vi "steuerprogramm.vi"() -> ()   [LabVIEW 2010]
uses:
  <vilib>/userDefined/High Color/nirio_resource_hc.ctl
  <vilib>/rvi/interface/nirviOpenFPGA/nirviOpenFPGA.xnode
  C:/Users/HAGAR-IV/Desktop/Zeugs/markus/version feb 2012/test/Auslesenkopiekopie2.vi
  <vilib>/rvi/interface/nirviMethod/nirviMethod.xnode
  <vilib>/rvi/interface/nirviReadWriteControl/nirviReadWriteControl.xnode
  <vilib>/rvi/errors/niLvFpgaWhatHappensToTopLevelVI.ctl
  <vilib>/rvi/interface/common/niFpgaNodeNameForErrorReporting.ctl
  <vilib>/rvi/errors/niLvFpgaAdjustHostInterfaceError.vi
  gvbooleschRT.vi
  <vilib>/functionblocks/FB Core/FB Core.xnode
  <vilib>/functionblocks/Counter/Elapsed Timer/Elapsed Timer.vi
  <vilib>/functionblocks/NI_FunctionBlock Libraries.lvlib
  <vilib>/rvi/interface/nirviCloseFPGA/nirviCloseFPGA.xnode
  <vilib>/addons/control/pid/NI_PID_pid.lvlib
  <vilib>/addons/control/pid/pid.llb/PID (DBL).vi
  <vilib>/LabVIEW Targets/FPGA/cRIO/shared/nicrio_ModuleControls/nicrio_cRIO-9871_BaudRateEnum.ctl
  <vilib>/LabVIEW Targets/FPGA/cRIO/shared/nicrio_ModuleControls/nicrio_cRIO-9871_DataBitsEnum.ctl
  <vilib>/LabVIEW Targets/FPGA/cRIO/shared/nicrio_ModuleControls/nicrio_cRIO-9871_ParityEnum.ctl
  <vilib>/LabVIEW Targets/FPGA/cRIO/shared/nicrio_ModuleControls/nicrio_cRIO-9871_StopBitsEnum.ctl
  <vilib>/LabVIEW Targets/FPGA/cRIO/shared/nicrio_ModuleControls/nicrio_cRIO-9871_FlowControlEnum.ctl
  <vilib>/addons/internet/NI_InternetTK_FTP_VIs.lvlib
  <vilib>/RVI Host/nirviSupport.llb/nirviErrorClusterFromErrorCode.vi
  <vilib>/FPGAPlugInAG/cRIO-9114/niLvFpga_Close_cRIO-9114.vi
panel:
  out "status":bool
  out "Array":dbl[](array[numeric])
  in  "nach sp warten(ms)":u32=10
  out "RS232 Array":string[](array[string])
  in  "Wartezeit nach MW(ms)":u32
  in  "Wartezeit nach SP(s)":dbl
  out "MFC1A Integriert":dbl
  in  "Eingang":T1(array[cluster])=[{"Zykluslängen [s]"=[120.0, 120.0, 120.0, 120.0], "ZeitpktDIOsMod0"=[0.0, 120.0], "ZeitpktDIOsMod1"=[0.0, 60.0, 62.0, 70.0, 120.0], "ZeitpktDIOsMod2A"=[0.0, 120.0], "ZeitpktDIOsMod2B"=[0.0, 60.0, 120.0], "DIOsSPMod0"=[[FALSE], [FALSE]], "DIOsSPMod1"=[[FALSE, FALSE, FALSE, FALSE, FALSE, TRUE, TRUE, FALSE, FALSE, FALSE, TRUE, FALSE, FALSE, FALSE, FALSE, FALSE, FALSE, FALSE], [FALSE, FALSE, FALSE, FALSE, FALSE, FALSE, TRUE, FALSE, FALSE, FALSE, FALSE, FALSE, FALSE, FALSE, FALSE, FALSE, TRUE, FALSE], [FALSE, FALSE, FALSE, FALSE, FALSE, FALSE, TRUE, FALSE, FALSE, FALSE, TRUE, FALSE, FALSE, FALSE, FALSE, FALSE, TRUE, FALSE], [FALSE, FALSE, FALSE, FALSE, FALSE, FALSE, TRUE, FALSE, FALSE, FALSE, TRUE, FALSE, FALSE, FALSE, FALSE, FALSE, FALSE, FALSE], [FALSE, FALSE, FALSE, FALSE, FALSE, FALSE, TRUE, FALSE, FALSE, FALSE, TRUE, FALSE, FALSE, FALSE, FALSE, FALSE, FALSE, FALSE]], "DIOsSPMod2A"=[[FALSE], [FALSE]], "DIOsSPMod2B"=[[FALSE], [FALSE]], "Mod0HorstZeitpkt"=[0.0, 120.0], "Mod1HorstZeitpkt"=[0.0, 59.0, 62.0, 120.0], "Mod2AHorstZeitpkt"=[0.0, 120.0], "Mod2BHorstZeitpkt"=[0.0, 120.0], "HorstSPMod0"=[[0.0], [0.0]], "HorstSPMod1"=[[3.0, 0.0, 0.8], [0.0, 0.0, 0.8], [1.0, 0.0, 0.8], [1.0, 0.0, 0.8]], "HorstSPMod2A"=[[0.0], [0.0]], "HorstSPMod2B"=[[0.0], [0.0]], "LangsameHeizungenSP"=[0.0, 100.0, 100.0, 0.0, 0.0, 0.0], "LHHeizen?"=[FALSE, TRUE, FALSE, FALSE, FALSE, FALSE], "ZPktFPGABoolesch"=[0.0, 62.0, 70.0, 120.0], "FPGABoolesch"=[[FALSE, FALSE, FALSE, FALSE, FALSE, FALSE], [FALSE, FALSE, TRUE, FALSE, FALSE, FALSE], [FALSE, FALSE, FALSE, FALSE, FALSE, FALSE], [FALSE, FALSE, FALSE, FALSE, FALSE, FALSE]], "ZeitpktFPGAPID"=[0.0, 120.0], "FPGAPID"=[[{"proportional gain (Kc)"=1.0, "integral gain (Kc*Ts/Ti)"=1.66796875, "derivative gain (Kc*Td/Ts)"=0.0}, {"proportional gain (Kc)"=1.0, "integral gain (Kc*Ts/Ti)"=1.66796875, "derivative gain (Kc*Td/Ts)"=0.0}, {"proportional gain (Kc)"=5.0, "integral gain (Kc*Ts/Ti)"=0.03515625, "derivative gain (Kc*Td/Ts)"=0.0234375}, {"proportional gain (Kc)"=1.0, "integral gain (Kc*Ts/Ti)"=1.66796875, "derivative gain (Kc*Td/Ts)"=0.0}], [{"proportional gain (Kc)"=1.0, "integral gain (Kc*Ts/Ti)"=1.66796875, "derivative gain (Kc*Td/Ts)"=0.0}, {"proportional gain (Kc)"=1.0, "integral gain (Kc*Ts/Ti)"=1.66796875, "derivative gain (Kc*Td/Ts)"=0.0}, {"proportional gain (Kc)"=5.0, "integral gain (Kc*Ts/Ti)"=0.03515625, "derivative gain (Kc*Td/Ts)"=0.0234375}, {"proportional gain (Kc)"=1.0, "integral gain (Kc*Ts/Ti)"=1.66796875, "derivative gain (Kc*Td/Ts)"=0.0}], [{"proportional gain (Kc)"=0.0, "integral gain (Kc*Ts/Ti)"=0.0, "derivative gain (Kc*Td/Ts)"=0.0}, {"proportional gain (Kc)"=0.0, "integral gain (Kc*Ts/Ti)"=0.0, "derivative gain (Kc*Td/Ts)"=0.0}, {"proportional gain (Kc)"=5.0, "integral gain (Kc*Ts/Ti)"=0.03125, "derivative gain (Kc*Td/Ts)"=0.01953125}, {"proportional gain (Kc)"=0.0, "integral gain (Kc*Ts/Ti)"=0.0, "derivative gain (Kc*Td/Ts)"=0.0}], [{"proportional gain (Kc)"=0.0, "integral gain (Kc*Ts/Ti)"=0.0, "derivative gain (Kc*Td/Ts)"=0.0}, {"proportional gain (Kc)"=0.0, "integral gain (Kc*Ts/Ti)"=0.0, "derivative gain (Kc*Td/Ts)"=0.0}, {"proportional gain (Kc)"=5.0, "integral gain (Kc*Ts/Ti)"=0.03125, "derivative gain (Kc*Td/Ts)"=0.01953125}, {"proportional gain (Kc)"=0.0, "integral gain (Kc*Ts/Ti)"=0.0, "derivative gain (Kc*Td/Ts)"=0.0}], [{"proportional gain (Kc)"=0.0, "integral gain (Kc*Ts/Ti)"=0.0, "derivative gain (Kc*Td/Ts)"=0.0}, {"proportional gain (Kc)"=0.0, "integral gain (Kc*Ts/Ti)"=0.0, "derivative gain (Kc*Td/Ts)"=0.0}, {"proportional gain (Kc)"=5.0, "integral gain (Kc*Ts/Ti)"=0.03125, "derivative gain (Kc*Td/Ts)"=0.01953125}, {"proportional gain (Kc)"=0.0, "integral gain (Kc*Ts/Ti)"=0.0, "derivative gain (Kc*Td/Ts)"=0.0}]], "ZeitpktFPGAFixp"=[0.0, 120.0], "FPGAFixp"=[[3.5, 3.5, 1.800048828125, 0.0, 0.0, 0.0, 2.400146484375, 0.0], [3.5, 3.5, 1.800048828125, 0.0, 0.0, 0.0, 2.400146484375, 0.0]], "ZeitpktMach1"=[0.0, 65.0, 72.0, 110.0, 111.0, 120.0], "TempMach1"=[70.0, 70.0, 150.0, 150.0, 70.0, 70.0], "ZeitpktMach2"=[0.0, 0.0, 120.0], "TempMach2"=[0.0, 0.0, 0.0], "PIDs für \"träge\" Heizungen"=[{"proportional gain (Kc)"=1.0, "integral time (Ti, min)"=0.01, "derivative time (Td, min)"=0.0}, {"proportional gain (Kc)"=5.0, "integral time (Ti, min)"=5.0, "derivative time (Td, min)"=5.0}, {"proportional gain (Kc)"=5.0, "integral time (Ti, min)"=1.0, "derivative time (Td, min)"=5.0}, {"proportional gain (Kc)"=1.0, "integral time (Ti, min)"=0.01, "derivative time (Td, min)"=0.0}, {"proportional gain (Kc)"=1.0, "integral time (Ti, min)"=0.01, "derivative time (Td, min)"=0.0}, {"proportional gain (Kc)"=1.0, "integral time (Ti, min)"=0.01, "derivative time (Td, min)"=0.0}], "Zwangsbedingungen"=[[0.0, 0.0, 0.0, 0.0, 0.0]], "Text0 MS-Datei"="text0", "Info"="info", "wie wird gespeichert?"=0, "Speicherlänge"="100", "Dateien fürs MS schicken?"=FALSE, "Pfad MS-Datei CRIO"=path "c:/"}] {"FPGAPID"."proportional gain (Kc)" format="%.11g"; "FPGAPID"."integral gain (Kc*Ts/Ti)" format="%.11g"; "FPGAPID"."derivative gain (Kc*Td/Ts)" format="%.11g"; "FPGAFixp" format="%.14g"}
  out "Ausgang":T2 {"FPGAPID"."proportional gain (Kc)" format="%.11g"; "FPGAPID"."integral gain (Kc*Ts/Ti)" format="%.11g"; "FPGAPID"."derivative gain (Kc*Td/Ts)" format="%.11g"; "FPGAFixp" format="%.14g"}
  out "Zykluslängen [s]":dbl[](array[numeric])
  in  "Tafel putzen1":bool
  in  "Tafel putzen2":bool
  in  "veränderte Methode benutzen":bool
  out "veränderte Methode":T2 {"FPGAPID"."proportional gain (Kc)" format="%.11g"; "FPGAPID"."integral gain (Kc*Ts/Ti)" format="%.11g"; "FPGAPID"."derivative gain (Kc*Td/Ts)" format="%.11g"; "FPGAFixp" format="%.14g"}
  in  "Methode verändern":bool
  in  "dargestellte Größe 2":i32(ring)=1 items=["T-MainCol3", "T-Trap1", "T-Trap2", "T-Stirling", "T-PreCol1", "T-PreCol2", "T-MainCol1", "T-MainCol2", "T-T-Line2", "T-MI1", "T-MI2", "T-MI3", "T-MI4", "T-MI5", "T-MI6", "F-MFM1", "T-MainCol4", "T-BHorst1", "T-BHorst2", "T-BHorst3", "T-BHorst4", "T-Oven1", "T-Oven2", "T-T-Line1", "F-MFM2", "P-Me-HP", "P-Me-LP", "P-Vac", "Ref-Turbo", "I-MS-AC", "I-Trap1", "I-Trap2", "Mod2/AI0", "Mod2/AI1", "Mod2/AI2", "Mod2/AI3", "Mod2/AI4", "Mod2/AI5", "Mod2/AI6", "Mod2/AI7", "Mod2/AI8", "Mod2/AI9", "Mod2/AI10", "Mod2/AI11", "Mod2/AI12", "Mod2/AI13", "Mod2/AI14", "Mod2/AI15", "Mod2/AI16", "Mod2/AI17", "Mod2/AI18", "Mod2/AI19", "Mod2/AI20", "Mod2/AI21", "Mod2/AI22", "Mod2/AI23", "Mod2/AI24", "Mod2/AI25", "Mod2/AI26", "Mod2/AI27", "Mod2/AI28", "Mod2/AI29", "Mod2/AI30", "Mod2/AI31", "Mod3/AI0", "Mod3/AI1", "Mod3/AI2", "Mod3/AI3", "Mod3/AI4", "Mod3/AI5", "Mod3/AI6", "Mod3/AI7", "Mod3/AI8", "Mod3/AI9", "Mod3/AI10", "Mod3/AI11", "Mod3/AI12", "Mod3/AI13", "Mod3/AI14", "Mod3/AI15", "Mod3/AI16", "Mod3/AI17", "Mod3/AI18", "Mod3/AI19", "Mod3/AI20", "Mod3/AI21", "Mod3/AI22", "Mod3/AI23", "Mod3/AI24", "Mod3/AI25", "Mod3/AI26", "Mod3/AI27", "Mod3/AI28", "Mod3/AI29", "Mod3/AI30", "Mod3/AI31", "U_Widr.Trap1 [V]", "Temp.Trap1 [°C]", "U_Widr.Trap2 [V]", "Temp.Trap2 [°C]", "Temp.Mach1 [°C]", "Temp.Mach2 [°C]", "MFC1B", "PressContr1A", "PressContr1B", "PressContr1C", "MFC1A", "PressContr1D", "MFC1A Integriert"]
  in  "Zeitachse2":i32(ring)=1 items=["Zykluszeit [s] Mod0", "Zykluszeit [s] Mod1", "Zykluszeit [s] Mod2A", "Zykluszeit [s] Mod2B"]
  out "Anzeige2":cluster{dbl[], dbl[]}(graph)
  out "Datum/Zeit":string
  in  "wie wird gespeichert?":u16(ring) items=["Time", "Cycle", "All"]
  out "Text 6":string
  in  "Info":string
  in  "Speicherlänge":string
  in  "Dateien fürs MS schicken?":bool
  in  "Pfad MS-Datei CRIO":path
  in  "Text0 MS-Datei":string
  out "ZwangsHorst!":cluster{dbl[]}[](array[cluster])
  out "ZwangsHorst?":cluster{bool[]}[](array[cluster])
  out "ZwangsDIO!":cluster{bool[]}[](array[cluster])
  out "ZwangsDIO?":cluster{bool[]}[](array[cluster])
  out "PIDs für \"träge\" Heizungen":T3(array[cluster])
  out "ZwangsLangsameH!":bool[](array[boolean])
  in  "Heizen?LH":bool[](array[boolean])
  out "Zwangsbedingungen":dbl[][](array[numeric])
  out "Traps/Machs":dbl[](array[numeric])
  out "ZwangsFPGABoolesch!":bool[](array[boolean])
  out "ZwangsFPGABoolesch?":bool[](array[boolean])
  in  "LangsameHeizungen%":u32[](array[numeric])
  in  "LangsameHeizungenSP":dbl[](array[numeric])
  out "ZwangsLangsameH?":bool[](array[boolean])
  out "Zykluszeiten 0, 1, 2A, 2B":dbl[](array[numeric])
  out "Zyklusnummern 0, 1, 2A, 2B":i32[](array[numeric])
  in  "dargestellte Größe 1":i32(ring)=1 items=["T-MainCol3", "T-Trap1", "T-Trap2", "T-Stirling", "T-PreCol1", "T-PreCol2", "T-MainCol1", "T-MainCol2", "T-T-Line2", "T-MI1", "T-MI2", "T-MI3", "T-MI4", "T-MI5", "T-MI6", "F-MFM1", "T-MainCol4", "T-BHorst1", "T-BHorst2", "T-BHorst3", "T-BHorst4", "T-Oven1", "T-Oven2", "T-T-Line1", "F-MFM2", "P-Me-HP", "P-Me-LP", "P-Vac", "Ref-Turbo", "I-MS-AC", "I-Trap1", "I-Trap2", "Mod2/AI0", "Mod2/AI1", "Mod2/AI2", "Mod2/AI3", "Mod2/AI4", "Mod2/AI5", "Mod2/AI6", "Mod2/AI7", "Mod2/AI8", "Mod2/AI9", "Mod2/AI10", "Mod2/AI11", "Mod2/AI12", "Mod2/AI13", "Mod2/AI14", "Mod2/AI15", "Mod2/AI16", "Mod2/AI17", "Mod2/AI18", "Mod2/AI19", "Mod2/AI20", "Mod2/AI21", "Mod2/AI22", "Mod2/AI23", "Mod2/AI24", "Mod2/AI25", "Mod2/AI26", "Mod2/AI27", "Mod2/AI28", "Mod2/AI29", "Mod2/AI30", "Mod2/AI31", "Mod3/AI0", "Mod3/AI1", "Mod3/AI2", "Mod3/AI3", "Mod3/AI4", "Mod3/AI5", "Mod3/AI6", "Mod3/AI7", "Mod3/AI8", "Mod3/AI9", "Mod3/AI10", "Mod3/AI11", "Mod3/AI12", "Mod3/AI13", "Mod3/AI14", "Mod3/AI15", "Mod3/AI16", "Mod3/AI17", "Mod3/AI18", "Mod3/AI19", "Mod3/AI20", "Mod3/AI21", "Mod3/AI22", "Mod3/AI23", "Mod3/AI24", "Mod3/AI25", "Mod3/AI26", "Mod3/AI27", "Mod3/AI28", "Mod3/AI29", "Mod3/AI30", "Mod3/AI31", "U_Widr.Trap1 [V]", "Temp.Trap1 [°C]", "U_Widr.Trap2 [V]", "Temp.Trap2 [°C]", "Temp.Mach1 [°C]", "Temp.Mach2 [°C]", "MFC1B", "PressContr1A", "PressContr1B", "PressContr1C", "MFC1A", "PressContr1D", "MFC1A Integriert"]
  in  "Zeitachse1":i32(ring)=1 items=["Zykluszeit [s] Mod0", "Zykluszeit [s] Mod1", "Zykluszeit [s] Mod2A", "Zykluszeit [s] Mod2B"]
  out "Anzeige1":cluster{dbl[], dbl[]}(graph)
  out "Big Ben, Methodenzeit, Zykluszeit0, Zykluszeit1, Zykluszeit2A, Zykluszeit2B":dbl[](array[numeric])
  out "MWHorst":dbl[](array[numeric])
  out "HorstSP":dbl[](array[numeric])
  out "RS-232":string
  out "Zähler serielle Kommunikation":i32
  out "Mod1Mod2Mod3/AITrapsMachs1Hz":dbl[](array[numeric])
  out "Mod3/AI":dbl[](array[numeric])
  out "Mod2/AI":dbl[](array[numeric])
  out "Mod1/AI":dbl[](array[numeric])
  in  "global stop RT":bool
  out "Big Ben":dbl
  out "Methodenzeit":dbl
  out "Zyklnum1ges":i32
  out "aktuelle TDMS-Datei":refnum<k34>
  in  "Methodennummer":i32(ring) items=["0"]
  out "Methodenwechsel?":bool
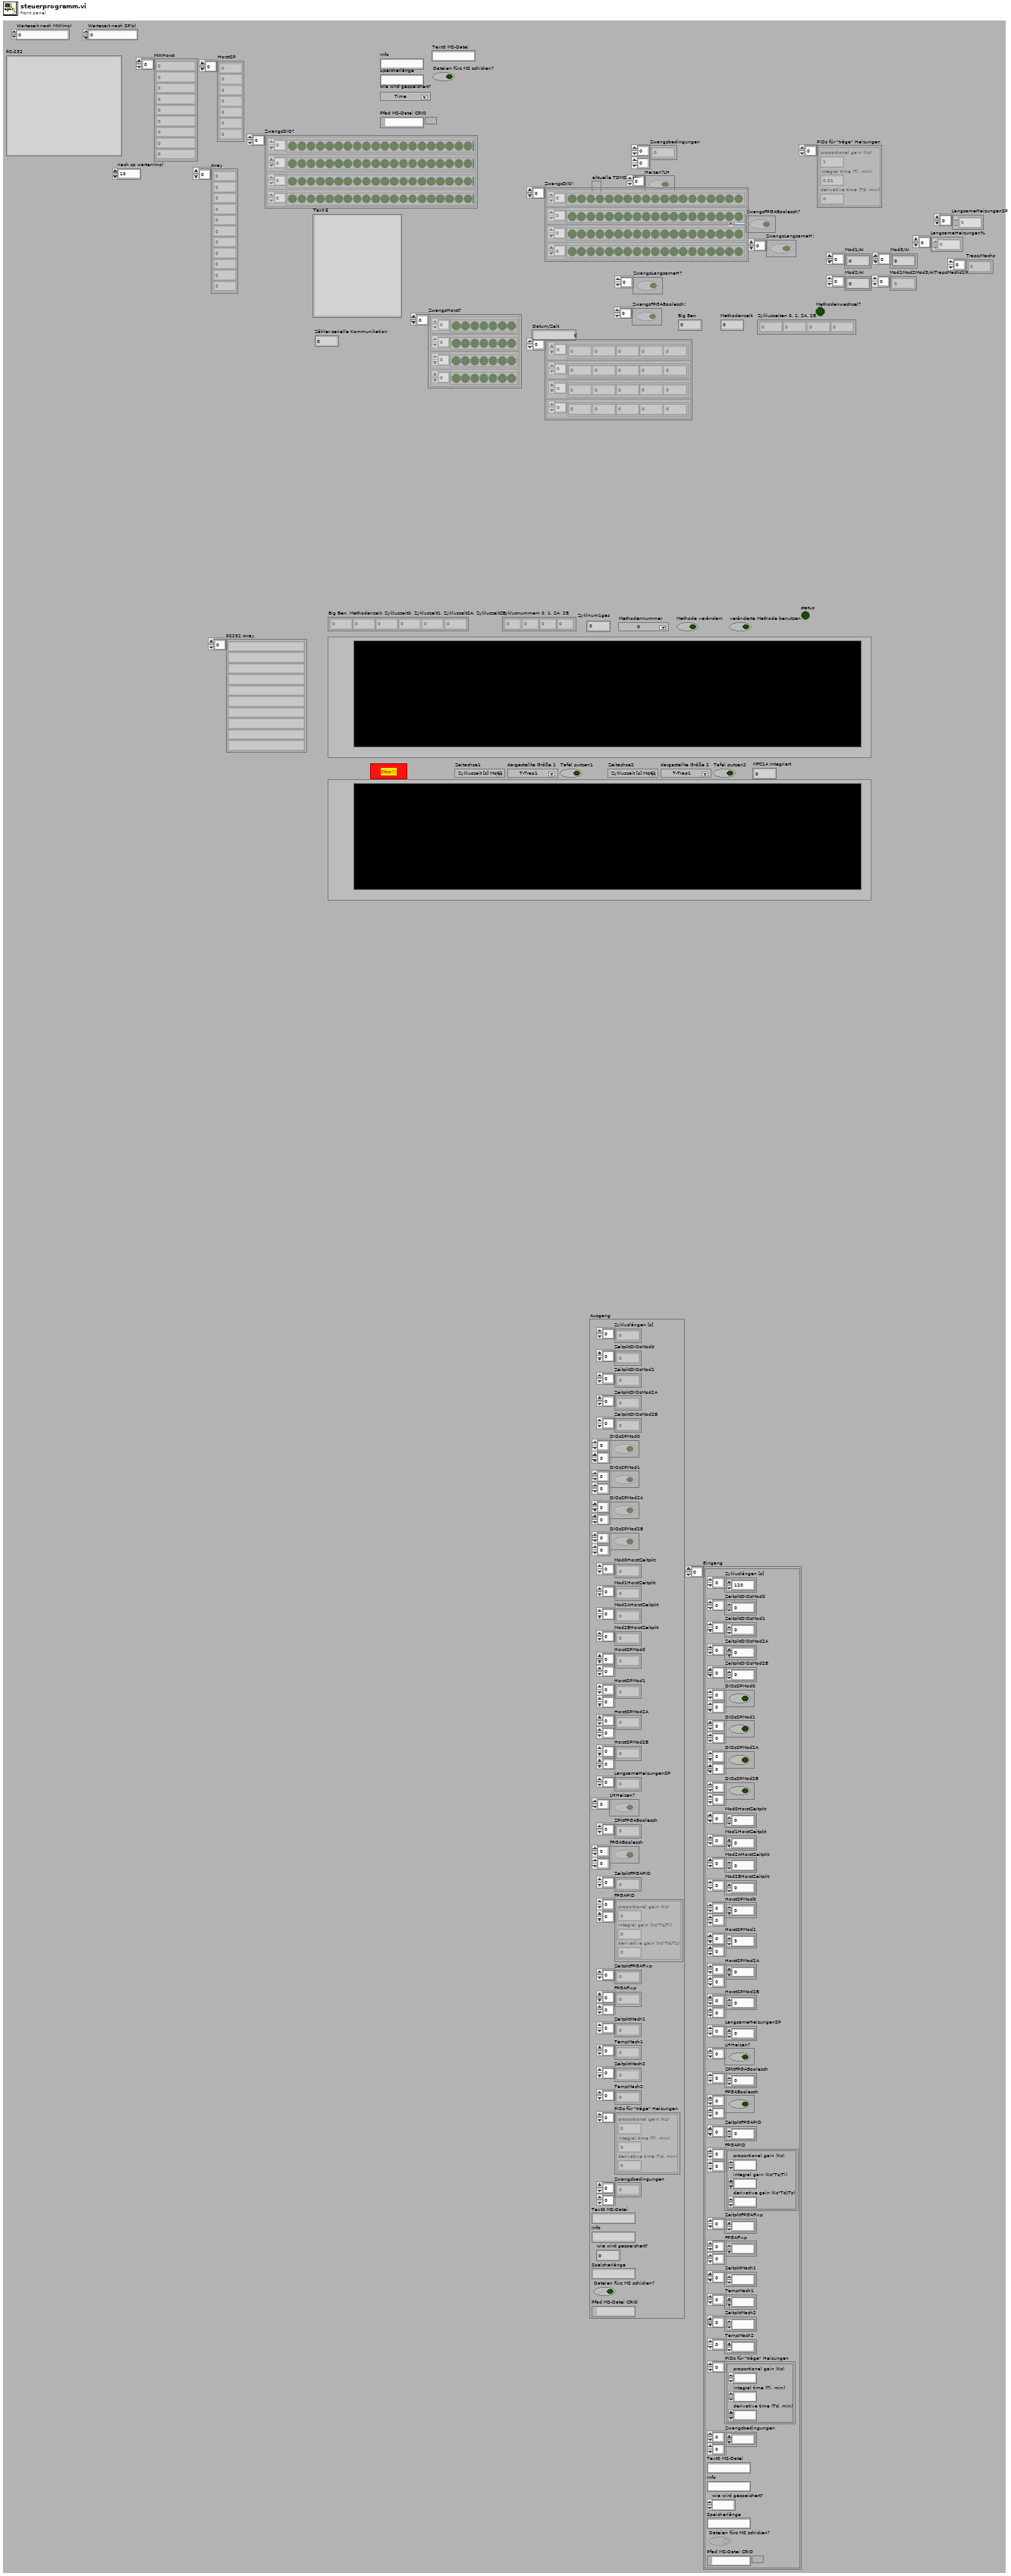
[diagram p1: front panel]
types:
  T1 = cluster{"Zykluslängen [s]":dbl[], "ZeitpktDIOsMod0":dbl[], "ZeitpktDIOsMod1":dbl[], "ZeitpktDIOsMod2A":dbl[], "ZeitpktDIOsMod2B":dbl[], "DIOsSPMod0":bool[][], "DIOsSPMod1":bool[][], "DIOsSPMod2A":bool[][], "DIOsSPMod2B":bool[][], "Mod0HorstZeitpkt":dbl[], "Mod1HorstZeitpkt":dbl[], "Mod2AHorstZeitpkt":dbl[], "Mod2BHorstZeitpkt":dbl[], "HorstSPMod0":dbl[][], "HorstSPMod1":dbl[][], "HorstSPMod2A":dbl[][], "HorstSPMod2B":dbl[][], "LangsameHeizungenSP":dbl[], "LHHeizen?":bool[], "ZPktFPGABoolesch":dbl[], "FPGABoolesch":bool[][], "ZeitpktFPGAPID":dbl[], "FPGAPID":cluster{"proportional gain (Kc)":fxp<+/-,16,8>, "integral gain (Kc*Ts/Ti)":fxp<+/-,16,8>, "derivative gain (Kc*Td/Ts)":fxp<+/-,16,8>}[][], "ZeitpktFPGAFixp":dbl[], "FPGAFixp":fxp<+/-,16,4>[][], "ZeitpktMach1":dbl[], "TempMach1":dbl[], "ZeitpktMach2":dbl[], "TempMach2":dbl[], "PIDs für \"träge\" Heizungen":cluster{"proportional gain (Kc)":dbl, "integral time (Ti, min)":dbl, "derivative time (Td, min)":dbl}[], "Zwangsbedingungen":dbl[][], "Text0 MS-Datei":string, "Info":string, "wie wird gespeichert?":u16, "Speicherlänge":string, "Dateien fürs MS schicken?":bool, "Pfad MS-Datei CRIO":path}[]
  T2 = cluster{"Zykluslängen [s]":dbl[], "ZeitpktDIOsMod0":dbl[], "ZeitpktDIOsMod1":dbl[], "ZeitpktDIOsMod2A":dbl[], "ZeitpktDIOsMod2B":dbl[], "DIOsSPMod0":bool[][], "DIOsSPMod1":bool[][], "DIOsSPMod2A":bool[][], "DIOsSPMod2B":bool[][], "Mod0HorstZeitpkt":dbl[], "Mod1HorstZeitpkt":dbl[], "Mod2AHorstZeitpkt":dbl[], "Mod2BHorstZeitpkt":dbl[], "HorstSPMod0":dbl[][], "HorstSPMod1":dbl[][], "HorstSPMod2A":dbl[][], "HorstSPMod2B":dbl[][], "LangsameHeizungenSP":dbl[], "LHHeizen?":bool[], "ZPktFPGABoolesch":dbl[], "FPGABoolesch":bool[][], "ZeitpktFPGAPID":dbl[], "FPGAPID":cluster{"proportional gain (Kc)":fxp<+/-,16,8>, "integral gain (Kc*Ts/Ti)":fxp<+/-,16,8>, "derivative gain (Kc*Td/Ts)":fxp<+/-,16,8>}[][], "ZeitpktFPGAFixp":dbl[], "FPGAFixp":fxp<+/-,16,4>[][], "ZeitpktMach1":dbl[], "TempMach1":dbl[], "ZeitpktMach2":dbl[], "TempMach2":dbl[], "PIDs für \"träge\" Heizungen":cluster{"proportional gain (Kc)":dbl, "integral time (Ti, min)":dbl, "derivative time (Td, min)":dbl}[], "Zwangsbedingungen":dbl[][], "Text0 MS-Datei":string, "Info":string, "wie wird gespeichert?":u16, "Speicherlänge":string, "Dateien fürs MS schicken?":bool, "Pfad MS-Datei CRIO":path}
  T3 = cluster{"proportional gain (Kc)":dbl, "integral time (Ti, min)":dbl, "derivative time (Td, min)":dbl}[]
  T4 = cluster{"DIOsMod0Nr":i32[], "DIOsMod1Nr":i32[], "DIOsMod2ANr":i32[], "DIOsMod2BNr":i32[], "AIs für \"träge\" Heizungen":i32[], i32[], "AnschlüsseHorstMod0":enum8{"0", "1", "2", "3", "4", "5", "6", "7", "8"}[], "AnschlüsseHorstMod1":enum8{"0", "1", "2", "3", "4", "5", "6", "7", "8"}[], "AnschlüsseHorstMod2A":enum8{"0", "1", "2", "3", "4", "5", "6", "7", "8"}[], "AnschlüsseHorstMod2B":enum8{"0", "1", "2", "3", "4", "5", "6", "7", "8"}[], "StringSPvorgebenMod0":string[], "StringSPvorgebenMod1":string[], "StringSPvorgebenMod2A":string[], "StringSPvorgebenMod2B":string[], "StringMWAntwort0":string[], "StringMWAntwort1":string[], "StringMWAntwort2A":string[], "StringMWAntwort2B":string[], "UmrechnungHorst0":dbl[], "UmrechnungHorst1":dbl[], "UmrechnungHorst2A":dbl[], "UmrechnungHorst2B":dbl[], "StringMWabfragenMod0":string[], "StringMWabfragenMod1":string[], "StringMWabfragenMod2A":string[], "StringMWabfragenMod2B":string[], "Modul1/AI koeff":dbl[][], "Modul2/AI koeff":dbl[][], "Modul3/AI koeff":dbl[][], "Traps/MachKoeff":dbl[][], "AIsNamen":string[], "DIOsMod0Name":string[], "DIOsMod1Name":string[], "DIOsMod2AName":string[], "DIOsMod2BName":string[], "HorstMod0Name":string[], "HorstMod1Name":string[], "HorstMod2AName":string[], "HorstMod2BName":string[], "Startmethode":i32, "Dateiordner Housekeeping":path, "Dateiname Housekeeping":string}
  T5 = enum16{"open", "open or create", "create or replace", "create", "open (read-only)"}
  T6 = enum16{"open", "replace", "create", "open or create", "replace or create", "replace or create with confirmation"}
  T7 = typedef "niFpgaNodeNameForErrorReporting.ctl" = enum16{"Open FPGA VI Reference", "Read/Write Control", "Invoke Method: Abort", "Invoke Method: Acknowledge IRQ", "Invoke Method: Download", "Invoke Method: FIFO.Configure", "Invoke Method: FIFO.Read", "Invoke Method: FIFO.Start", "Invoke Method: FIFO.Stop", "Invoke Method: FIFO.Write", "Invoke Method: Reset", "Invoke Method: Run", "Invoke Method: Wait on IRQ", "Close FPGA VI Reference"}
  T8 = typedef "niLvFpgaWhatHappensToTopLevelVI.ctl" = enum16{"top level VI scripted behind XNode", "top level VI inlined behind XNode"}
  T9 = enum8{"0", "1", "2", "3", "4", "5", "6", "7", "8"}
  T10 = typedef "nicrio_cRIO-9871_BaudRateEnum.ctl" = enum16{"75 bps", "110 bps", "134 bps", "150 bps", "300 bps", "600 bps", "1200 bps", "1800 bps", "2400 bps", "4800 bps", "7200 bps", "9600 bps", "14.4 kbps", "19.2 kbps", "28.8 kbps", "38.4 kbps", "57.6 kbps", "115.2 kbps", "230.4 kbps", "460.8 kbps", "921.6 kbps"}
  T11 = typedef "nicrio_cRIO-9871_DataBitsEnum.ctl" = enum8{"5", "6", "7", "8"}
  T12 = typedef "nicrio_cRIO-9871_ParityEnum.ctl" = enum8{"None", "Odd", "Even", "Mark", "Space"}
  T13 = typedef "nicrio_cRIO-9871_StopBitsEnum.ctl" = enum8{"1", "1.5", "2"}
  T14 = typedef "nicrio_cRIO-9871_FlowControlEnum.ctl" = enum8{"None", "Software (XON / XOFF)", "Hardware (RTS / CTS)"}
  T15 = cluster{"Baud Rate":T10, "Data Bits":T11, "Parity":T12, "Stop Bits":T13, "Flow Control":T14}
  T16 = enum8{"0", "1", "2", "3", "4", "5", "6", "7", "8"}[]
  T17 = cluster{"DIOsMod0Name":string[], "DIOsMod1Name":string[], "DIOsMod2AName":string[], "DIOsMod2BName":string[], "HorstMod0Name":string[], "HorstMod1Name":string[], "HorstMod2AName":string[], "HorstMod2BName":string[], string[]}
  T18 = cluster{"PIDs für \"träge\" Heizungen[0]":cluster{"proportional gain (Kc)":dbl, "integral time (Ti, min)":dbl, "derivative time (Td, min)":dbl}, "PIDs für \"träge\" Heizungen[1]":cluster{"proportional gain (Kc)":dbl, "integral time (Ti, min)":dbl, "derivative time (Td, min)":dbl}, "PIDs für \"träge\" Heizungen[2]":cluster{"proportional gain (Kc)":dbl, "integral time (Ti, min)":dbl, "derivative time (Td, min)":dbl}, "PIDs für \"träge\" Heizungen[3]":cluster{"proportional gain (Kc)":dbl, "integral time (Ti, min)":dbl, "derivative time (Td, min)":dbl}, "PIDs für \"träge\" Heizungen[4]":cluster{"proportional gain (Kc)":dbl, "integral time (Ti, min)":dbl, "derivative time (Td, min)":dbl}, "PIDs für \"träge\" Heizungen[5]":cluster{"proportional gain (Kc)":dbl, "integral time (Ti, min)":dbl, "derivative time (Td, min)":dbl}}
  T19 = cluster{"LangsameHeizungenSP[0]":dbl, "LangsameHeizungenSP[1]":dbl, "LangsameHeizungenSP[2]":dbl, "LangsameHeizungenSP[3]":dbl, "LangsameHeizungenSP[4]":dbl, "LangsameHeizungenSP[5]":dbl}
  T20 = cluster{"[0]":dbl, "[1]":dbl, "[2]":dbl, "[3]":dbl, "[4]":dbl, "[5]":dbl}
  T21 = cluster{"proportional gain (Kc)":dbl, "integral time (Ti, min)":dbl, "derivative time (Td, min)":dbl}
  T22 = cluster{"Heizen?LH[0]":bool, "Heizen?LH[1]":bool, "Heizen?LH[2]":bool, "Heizen?LH[3]":bool, "Heizen?LH[4]":bool, "Heizen?LH[5]":bool}
  T23 = cluster{"LangsameHeizungen%[0]":u32, "LangsameHeizungen%[1]":u32, "LangsameHeizungen%[2]":u32, "LangsameHeizungen%[3]":u32, "LangsameHeizungen%[4]":u32, "LangsameHeizungen%[5]":u32}
  T24 = cluster{"Zykluslängen [s]":dbl[], "ZeitpktDIOsMod0":dbl[], "ZeitpktDIOsMod1":dbl[], "ZeitpktDIOsMod2A":dbl[], "ZeitpktDIOsMod2B":dbl[], "DIOsSPMod0":bool[][], "DIOsSPMod1":bool[][], "DIOsSPMod2A":bool[][], "DIOsSPMod2B":bool[][], "Mod0HorstZeitpkt":dbl[], "Mod1HorstZeitpkt":dbl[], "Mod2AHorstZeitpkt":dbl[], "Mod2BHorstZeitpkt":dbl[], "HorstSPMod0":dbl[][], "HorstSPMod1":dbl[][], "HorstSPMod2A":dbl[][], "HorstSPMod2B":dbl[][], "LangsameHeizungenSP":dbl[], "LHHeizen?":bool[], "ZPktFPGABoolesch":dbl[], "FPGABoolesch":bool[][], "ZeitpktFPGAPID":dbl[], "FPGAPID":cluster{"proportional gain (Kc)":fxp<+/-,16,8>, "integral gain (Kc*Ts/Ti)":fxp<+/-,16,8>, "derivative gain (Kc*Td/Ts)":fxp<+/-,16,8>}[][], "ZeitpktFPGAFixp":dbl[], "FPGAFixp":fxp<+/-,16,4>[][], "ZeitpktMach1":dbl[], "TempMach1":dbl[], "ZeitpktMach2":dbl[], "TempMach2":dbl[], "PIDs für \"träge\" Heizungen":cluster{"proportional gain (Kc)":dbl, "integral time (Ti, min)":dbl, "derivative time (Td, min)":dbl}[], "Zwangsbedingungen":dbl[][], "Dateien fürs MS schicken?":bool, "ZeitpunkteMPV":dbl[], "SPMPV":i32[], "ZeitpktMSa":dbl, "ZeitpktMSb":dbl, "Int.Start1":dbl, "Int.Stop1":dbl, "Int.Start2":dbl, "Int.Stop2":dbl, "Methodenname":string}
  T25 = cluster{"proportional gain (Kc)":fxp<+/-,16,8>, "integral gain (Kc*Ts/Ti)":fxp<+/-,16,8>, "derivative gain (Kc*Td/Ts)":fxp<+/-,16,8>}[][]
  T26 = cluster{"FPGAFixp[0]":fxp<+/-,16,4>, "FPGAFixp[1]":fxp<+/-,16,4>, "FPGAFixp[2]":fxp<+/-,16,4>, "FPGAFixp[3]":fxp<+/-,16,4>, "FPGAFixp[4]":fxp<+/-,16,4>, "FPGAFixp[5]":fxp<+/-,16,4>, "FPGAFixp[6]":fxp<+/-,16,4>, "FPGAFixp[7]":fxp<+/-,16,4>}
  T27 = cluster{"proportional gain (Kc)":fxp<+/-,16,8>, "integral gain (Kc*Ts/Ti)":fxp<+/-,16,8>, "derivative gain (Kc*Td/Ts)":fxp<+/-,16,8>}[]
  T28 = cluster{"FPGAPID[0]":cluster{"proportional gain (Kc)":fxp<+/-,16,8>, "integral gain (Kc*Ts/Ti)":fxp<+/-,16,8>, "derivative gain (Kc*Td/Ts)":fxp<+/-,16,8>}, "FPGAPID[1]":cluster{"proportional gain (Kc)":fxp<+/-,16,8>, "integral gain (Kc*Ts/Ti)":fxp<+/-,16,8>, "derivative gain (Kc*Td/Ts)":fxp<+/-,16,8>}, "FPGAPID[2]":cluster{"proportional gain (Kc)":fxp<+/-,16,8>, "integral gain (Kc*Ts/Ti)":fxp<+/-,16,8>, "derivative gain (Kc*Td/Ts)":fxp<+/-,16,8>}, "FPGAPID[3]":cluster{"proportional gain (Kc)":fxp<+/-,16,8>, "integral gain (Kc*Ts/Ti)":fxp<+/-,16,8>, "derivative gain (Kc*Td/Ts)":fxp<+/-,16,8>}}
  T29 = cluster{"proportional gain (Kc)":fxp<+/-,16,8>, "integral gain (Kc*Ts/Ti)":fxp<+/-,16,8>, "derivative gain (Kc*Td/Ts)":fxp<+/-,16,8>}
  T30 = cluster{"[0]":bool, "[1]":bool, "[2]":bool, "[3]":bool, "[4]":bool, "[5]":bool}
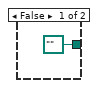
[diagram p2: hidden frame]
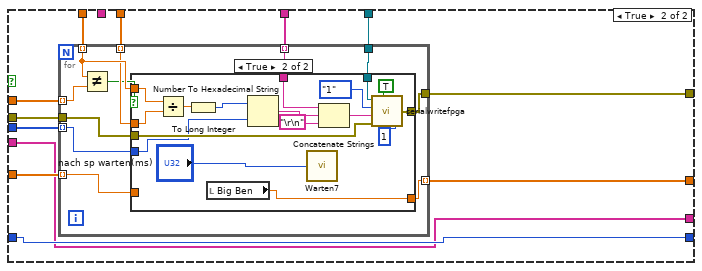
[diagram p4: hidden frame]
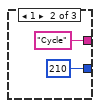
[diagram p8: hidden frame]
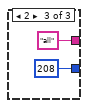
[diagram p9: hidden frame]
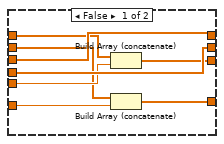
[diagram p12: hidden frame]
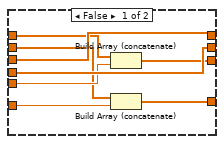
[diagram p13: hidden frame]
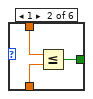
[diagram p16: hidden frame]
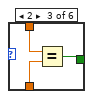
[diagram p17: hidden frame]
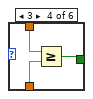
[diagram p18: hidden frame]
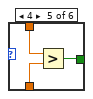
[diagram p19: hidden frame]
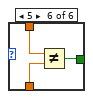
[diagram p20: hidden frame]
diagram:
  (unwired) T1 [{"Zykluslängen [s]"=[180.0, 180.0, 180.0, 180.0], "ZeitpktDIOsMod0"=[0.0, 180.0], "ZeitpktDIOsMod1"=[0.0, 2.0, 15.0, 60.0, 61.0, 70.0, 80.0, 170.0, 180.0], "ZeitpktDIOsMod2A"=[0.0, 180.0], "ZeitpktDIOsMod2B"=[0.0, 60.0, 180.0], "DIOsSPMod0"=[[FALSE], [FALSE]], "DIOsSPMod1"=[[TRUE, TRUE, FALSE, TRUE, FALSE, TRUE, TRUE, TRUE, FALSE, FALSE, TRUE, FALSE, FALSE, FALSE, FALSE, FALSE, FALSE, TRUE], [TRUE, FALSE, FALSE, TRUE, FALSE, TRUE, TRUE, TRUE, FALSE, FALSE, TRUE, FALSE, FALSE, FALSE, FALSE, FALSE, FALSE, TRUE], [TRUE, FALSE, FALSE, FALSE, FALSE, TRUE, TRUE, FALSE, FALSE, FALSE, TRUE, FALSE, FALSE, FALSE, FALSE, FALSE, TRUE, TRUE], [TRUE, FALSE, FALSE, FALSE, FALSE, FALSE, TRUE, FALSE, FALSE, FALSE, TRUE, FALSE, FALSE, FALSE, FALSE, FALSE, TRUE, TRUE], [TRUE, FALSE, FALSE, FALSE, FALSE, FALSE, TRUE, FALSE, FALSE, FALSE, TRUE, FALSE, FALSE, FALSE, FALSE, FALSE, TRUE, TRUE], [TRUE, FALSE, FALSE, FALSE, FALSE, FALSE, TRUE, FALSE, FALSE, FALSE, TRUE, FALSE, FALSE, FALSE, FALSE, FALSE, TRUE, TRUE], [TRUE, FALSE, FALSE, FALSE, FALSE, FALSE, TRUE, FALSE, FALSE, FALSE, TRUE, FALSE, FALSE, FALSE, FALSE, FALSE, FALSE, TRUE], [TRUE, FALSE, FALSE, FALSE, FALSE, FALSE, TRUE, FALSE, FALSE, FALSE, TRUE, FALSE, FALSE, FALSE, FALSE, FALSE, FALSE, TRUE], [TRUE, FALSE, FALSE, FALSE, FALSE, FALSE, TRUE, FALSE, FALSE, FALSE, TRUE, FALSE, FALSE, FALSE, FALSE, FALSE, FALSE, TRUE]], "DIOsSPMod2A"=[[FALSE], [FALSE]], "DIOsSPMod2B"=[[FALSE], [FALSE]], "Mod0HorstZeitpkt"=[0.0, 180.0], "Mod1HorstZeitpkt"=[0.0, 55.0, 75.0, 180.0], "Mod2AHorstZeitpkt"=[0.0, 20.0, 180.0], "Mod2BHorstZeitpkt"=[0.0, 380.0], "HorstSPMod0"=[[2.66], [2.66]], "HorstSPMod1"=[[1.9, 0.0, 1.2], [0.0, 0.0, 1.2], [1.9, 0.0, 1.2], [1.9, 0.0, 1.2]], "HorstSPMod2A"=[[300.0], [300.0], [300.0]], "HorstSPMod2B"=[[0.0], [0.0]], "LangsameHeizungenSP"=[60.0, 220.0, 120.0, 60.0, 110.0, 0.0], "LHHeizen?"=[FALSE, TRUE, TRUE, FALSE, TRUE, FALSE], "ZPktFPGABoolesch"=[0.0, 60.0, 75.0, 180.0], "FPGABoolesch"=[[FALSE, FALSE, FALSE, FALSE, TRUE, FALSE], [FALSE, FALSE, TRUE, FALSE, TRUE, FALSE], [FALSE, FALSE, FALSE, FALSE, TRUE, FALSE], [FALSE, FALSE, FALSE, FALSE, TRUE, FALSE]], "ZeitpktFPGAPID"=[0.0, 60.0, 180.0], "FPGAPID"=[[{"proportional gain (Kc)"=5.0, "integral gain (Kc*Ts/Ti)"=0.0, "derivative gain (Kc*Td/Ts)"=0.0}, {"proportional gain (Kc)"=1.0, "integral gain (Kc*Ts/Ti)"=1.66796875, "derivative gain (Kc*Td/Ts)"=0.0}, {"proportional gain (Kc)"=5.0, "integral gain (Kc*Ts/Ti)"=0.03515625, "derivative gain (Kc*Td/Ts)"=0.0234375}, {"proportional gain (Kc)"=1.0, "integral gain (Kc*Ts/Ti)"=1.66796875, "derivative gain (Kc*Td/Ts)"=0.0}], [{"proportional gain (Kc)"=5.0, "integral gain (Kc*Ts/Ti)"=0.0, "derivative gain (Kc*Td/Ts)"=0.0}, {"proportional gain (Kc)"=1.0, "integral gain (Kc*Ts/Ti)"=1.66796875, "derivative gain (Kc*Td/Ts)"=0.0}, {"proportional gain (Kc)"=5.0, "integral gain (Kc*Ts/Ti)"=0.03515625, "derivative gain (Kc*Td/Ts)"=0.0234375}, {"proportional gain (Kc)"=1.0, "integral gain (Kc*Ts/Ti)"=1.66796875, "derivative gain (Kc*Td/Ts)"=0.0}], [{"proportional gain (Kc)"=0.0, "integral gain (Kc*Ts/Ti)"=0.0, "derivative gain (Kc*Td/Ts)"=0.0}, {"proportional gain (Kc)"=0.0, "integral gain (Kc*Ts/Ti)"=0.0, "derivative gain (Kc*Td/Ts)"=0.0}, {"proportional gain (Kc)"=2.0, "integral gain (Kc*Ts/Ti)"=0.03125, "derivative gain (Kc*Td/Ts)"=0.01953125}, {"proportional gain (Kc)"=0.0, "integral gain (Kc*Ts/Ti)"=0.0, "derivative gain (Kc*Td/Ts)"=0.0}], [{"proportional gain (Kc)"=0.0, "integral gain (Kc*Ts/Ti)"=0.0, "derivative gain (Kc*Td/Ts)"=0.0}, {"proportional gain (Kc)"=0.0, "integral gain (Kc*Ts/Ti)"=0.0, "derivative gain (Kc*Td/Ts)"=0.0}, {"proportional gain (Kc)"=2.0, "integral gain (Kc*Ts/Ti)"=0.03125, "derivative gain (Kc*Td/Ts)"=0.01953125}, {"proportional gain (Kc)"=0.0, "integral gain (Kc*Ts/Ti)"=0.0, "derivative gain (Kc*Td/Ts)"=0.0}], [{"proportional gain (Kc)"=0.0, "integral gain (Kc*Ts/Ti)"=0.0, "derivative gain (Kc*Td/Ts)"=0.0}, {"proportional gain (Kc)"=0.0, "integral gain (Kc*Ts/Ti)"=0.0, "derivative gain (Kc*Td/Ts)"=0.0}, {"proportional gain (Kc)"=2.0, "integral gain (Kc*Ts/Ti)"=0.03125, "derivative gain (Kc*Td/Ts)"=0.01953125}, {"proportional gain (Kc)"=0.0, "integral gain (Kc*Ts/Ti)"=0.0, "derivative gain (Kc*Td/Ts)"=0.0}]], "ZeitpktFPGAFixp"=[0.0, 60.0, 75.0, 180.0], "FPGAFixp"=[[0.0, 0.0, 0.0, 0.0, 0.0, 0.0, 2.85009765625, 0.0], [4.59423828125, 4.599365234375, 1.699951171875, 0.0, 0.0, 0.0, 2.85009765625, 0.0], [0.0, 0.0, 0.0, 0.0, 0.0, 0.0, 2.85009765625, 0.0], [0.0, 0.0, 0.0, 0.0, 0.0, 0.0, 2.85009765625, 0.0]], "ZeitpktMach1"=[0.0, 1.0, 100.0, 101.0, 177.0, 178.0, 180.0], "TempMach1"=[50.0, 50.0, 50.0, 250.0, 250.0, 50.0, 50.0], "ZeitpktMach2"=[0.0, 0.0, 120.0], "TempMach2"=[0.0, 0.0, 0.0], "PIDs für \"träge\" Heizungen"=[{"proportional gain (Kc)"=1.0, "integral time (Ti, min)"=0.01, "derivative time (Td, min)"=0.0}, {"proportional gain (Kc)"=2.0, "integral time (Ti, min)"=1.0, "derivative time (Td, min)"=0.0}, {"proportional gain (Kc)"=4.0, "integral time (Ti, min)"=1.0, "derivative time (Td, min)"=0.0}, {"proportional gain (Kc)"=1.0, "integral time (Ti, min)"=0.01, "derivative time (Td, min)"=0.0}, {"proportional gain (Kc)"=2.0, "integral time (Ti, min)"=0.0, "derivative time (Td, min)"=0.0}, {"proportional gain (Kc)"=1.0, "integral time (Ti, min)"=0.01, "derivative time (Td, min)"=0.0}], "Zwangsbedingungen"=[[3.0, 4.0, 100.0, 23.0, 4.0, 200.0, 0.0, 0.0]], "Text0 MS-Datei"="text0", "Info"="info", "wie wird gespeichert?"=0, "Speicherlänge"="100", "Dateien fürs MS schicken?"=FALSE, "Pfad MS-Datei CRIO"=path "c:/"}] ("Eingang 2")
  (unwired) T4 {"DIOsMod0Nr"=[32], "DIOsMod1Nr"=[5, 6, 7, 10, 11, 14, 15, 16, 17, 18, 20, 23, 25, 26, 27, 28, 29, 30], "DIOsMod2ANr"=[33], "DIOsMod2BNr"=[34], "AIs für \"träge\" Heizungen"=[17, 6, 0, 19, 21, 23], [1, 3, 1, 1], "AnschlüsseHorstMod0"=[enum."1"], "AnschlüsseHorstMod1"=[enum."1", enum."1", enum."1"], "AnschlüsseHorstMod2A"=[enum."1"], "AnschlüsseHorstMod2B"=[enum."1"], "StringSPvorgebenMod0"=[":060A020121"], "StringSPvorgebenMod1"=[":060B020121", ":0618020121", ":060D020121"], "StringSPvorgebenMod2A"=[":0619020121"], "StringSPvorgebenMod2B"=[":060C020121"], "StringMWAntwort0"=[":060A020121"], "StringMWAntwort1"=[":060B020121", ":0618020121", ":060D020121"], "StringMWAntwort2A"=[":0619020121"], "StringMWAntwort2B"=[":060C020121"], "UmrechnungHorst0"=[0.0003125], "UmrechnungHorst1"=[9.375e-05, 9.375e-05, 9.375e-05], "UmrechnungHorst2A"=[0.046875], "UmrechnungHorst2B"=[9.375e-05], "StringMWabfragenMod0"=[":060A0401210120"], "StringMWabfragenMod1"=[":060B0401210120", ":06180401210120", ":060D0401210120"], "StringMWabfragenMod2A"=[":06190401210120"], "StringMWabfragenMod2B"=[":060C0401210120"], "Modul1/AI koeff"=[[-249.333, 111.873, 2.1471], [-249.333, 111.873, 2.1471], [-249.333, 111.873, 2.1471], [-249.333, 111.873, 2.1471], [-237.2852, -153.162, 6.0782], [-237.2852, -153.162, 6.0782], [-249.333, 111.873, 2.1471], [-249.333, 111.873, 2.1471], [-249.333, 111.873, 2.1471], [-249.333, 111.873, 2.1471], [-249.333, 111.873, 2.1471], [-249.333, 111.873, 2.1471], [-249.333, 111.873, 2.1471], [-249.333, 111.873, 2.1471], [-249.333, 111.873, 2.1471], [0.0, 1.0, 0.0], [-249.333, 111.873, 2.1471], [-249.333, 111.873, 2.1471], [-249.333, 111.873, 2.1471], [-249.333, 111.873, 2.1471], [-249.333, 111.873, 2.1471], [-249.333, 111.873, 2.1471], [-249.333, 111.873, 2.1471], [-249.333, 111.873, 2.1471], [0.0, 1.0, 0.0], [0.0, 1.0, 0.0], [0.0, 1.0, 0.0], [0.0, 1.0, 0.0], [0.0, 1.0, 0.0], [0.0, 1.0, 0.0], [0.0, 1.0, 0.0], [0.0, 1.0, 0.0]], "Modul2/AI koeff"=[[0.0, 1.0, 0.0], [0.0, 1.0, 0.0], [0.0, 1.0, 0.0], [0.0, 1.0, 0.0], [0.0, 1.0, 0.0], [0.0, 1.0, 0.0], [0.0, 1.0, 0.0], [0.0, 1.0, 0.0], [0.0, 1.0, 0.0], [0.0, 1.0, 0.0], [0.0, 1.0, 0.0], [0.0, 1.0, 0.0], [0.0, 1.0, 0.0], [0.0, 1.0, 0.0], [0.0, 1.0, 0.0], [0.0, 1.0, 0.0], [0.0, 1.0, 0.0], [0.0, 1.0, 0.0], [0.0, 1.0, 0.0], [0.0, 1.0, 0.0], [0.0, 1.0, 0.0], [0.0, 1.0, 0.0], [0.0, 1.0, 0.0], [0.0, 1.0, 0.0], [0.0, 1.0, 0.0], [0.0, 1.0, 0.0], [0.0, 1.0, 0.0], [0.0, 1.0, 0.0], [0.0, 1.0, 0.0], [0.0, 1.0, 0.0], [0.0, 1.0, 0.0], [0.0, 1.0, 0.0]], "Modul3/AI koeff"=[[0.0, 1.0, 0.0], [0.0, 1.0, 0.0], [0.0, 1.0, 0.0], [0.0, 1.0, 0.0], [0.0, 1.0, 0.0], [0.0, 1.0, 0.0], [0.0, 1.0, 0.0], [0.0, 1.0, 0.0], [0.0, 1.0, 0.0], [0.0, 1.0, 0.0], [0.0, 1.0, 0.0], [0.0, 1.0, 0.0], [0.0, 1.0, 0.0], [0.0, 1.0, 0.0], [0.0, 1.0, 0.0], [0.0, 1.0, 0.0], [0.0, 1.0, 0.0], [0.0, 1.0, 0.0], [0.0, 1.0, 0.0], [0.0, 1.0, 0.0], [0.0, 1.0, 0.0], [0.0, 1.0, 0.0], [0.0, 1.0, 0.0], [0.0, 1.0, 0.0], [0.0, 1.0, 0.0], [0.0, 1.0, 0.0], [0.0, 1.0, 0.0], [0.0, 1.0, 0.0], [0.0, 1.0, 0.0], [0.0, 1.0, 0.0], [0.0, 1.0, 0.0], [0.0, 1.0, 0.0]], "Traps/MachKoeff"=[[0.0, 1.0, 0.0], [-249.333, 111.873, 2.1471], [0.0, 1.0, 0.0], [-249.333, 111.873, 2.1471], [-237.2852, 153.1621, 6.0782], [-237.2852, 153.1621, 6.0782]], "AIsNamen"=["T-MainCol3", "T-Trap1", "T-Trap2", "T-Stirling", "T-PreCol1", "T-PreCol2", "T-MainCol1", "T-MainCol2", "T-T-Line2", "T-MI1", "T-MI2", "T-MI3", "T-MI4", "T-MI5", "T-MI6", "F-MFM1", "T-MainCol4", "T-BHorst1", "T-BHorst2", "T-BHorst3", "T-BHorst4", "T-Oven1", "T-Oven2", "T-T-Line1", "F-MFM2", "P-Me-HP", "P-Me-LP", "P-Vac", "Ref-Turbo", "I-MS-AC", "I-Trap1", "I-Trap2", "Mod2/AI0", "Mod2/AI1", "Mod2/AI2", "Mod2/AI3", "Mod2/AI4", "Mod2/AI5", "Mod2/AI6", "Mod2/AI7", "Mod2/AI8", "Mod2/AI9", "Mod2/AI10", "Mod2/AI11", "Mod2/AI12", "Mod2/AI13", "Mod2/AI14", "Mod2/AI15", "Mod2/AI16", "Mod2/AI17", "Mod2/AI18", "Mod2/AI19", "Mod2/AI20", "Mod2/AI21", "Mod2/AI22", "Mod2/AI23", "Mod2/AI24", "Mod2/AI25", "Mod2/AI26", "Mod2/AI27", "Mod2/AI28", "Mod2/AI29", "Mod2/AI30", "Mod2/AI31", "Mod3/AI0", "Mod3/AI1", "Mod3/AI2", "Mod3/AI3", "Mod3/AI4", "Mod3/AI5", "Mod3/AI6", "Mod3/AI7", "Mod3/AI8", "Mod3/AI9", "Mod3/AI10", "Mod3/AI11", "Mod3/AI12", "Mod3/AI13", "Mod3/AI14", "Mod3/AI15", "Mod3/AI16", "Mod3/AI17", "Mod3/AI18", "Mod3/AI19", "Mod3/AI20", "Mod3/AI21", "Mod3/AI22", "Mod3/AI23", "Mod3/AI24", "Mod3/AI25", "Mod3/AI26", "Mod3/AI27", "Mod3/AI28", "Mod3/AI29", "Mod3/AI30", "Mod3/AI31"], "DIOsMod0Name"=["blindDIO0"], "DIOsMod1Name"=["on/off P-MS", "MS Start", "MS Stop", "FanMach1", "FanReserve", "Valve1A", "on/off PrePump", "S1Reserve", "on/off VacP2", "on/off VacP1", "S1D", "FanMach2", "S1C", "on/off Stirling", "S1B", "S1A", "Valve1B", "on/off Turbo"], "DIOsMod2AName"=["blindDIO2A"], "DIOsMod2BName"=["blindDIO2B"], "HorstMod0Name"=["MFC1B"], "HorstMod1Name"=["PressContr1A", "PressContr1B", "PressContr1C"], "HorstMod2AName"=["MFC1A"], "HorstMod2BName"=["PressContr1D"], "Startmethode"=0, "Dateiordner Housekeeping"=path "C:/", "Dateiname Housekeeping"="test"} ("Einstellungen")
  n1 = flat-sequence {
    tunnel: [w113] -> w34
    tunnel: [w54] -> w33
    tunnel: [w124] -> w32
    tunnel: [w125] -> w31
    tunnel: [w112] -> w27
    tunnel: [w89] -> w26
    tunnel: [w63] -> w25
    tunnel: [w103] -> w24
    tunnel: [w74] -> w23
    tunnel: [w94] -> w22
    tunnel: [w88] -> w21
    tunnel: [w87] -> w20
    tunnel: [w86] -> w19
    tunnel: [w109] -> w18
    tunnel: [w85] -> w17
    tunnel: [w68] -> w16
    tunnel: [w62] -> w15
    tunnel: [w36] -> w14
    tunnel: [w111] -> w13
    tunnel: [w108] -> w12
    tunnel: [w108] -> w11
    tunnel: T4 {"DIOsMod0Nr"=[32], "DIOsMod1Nr"=[5, 6, 7, 10, 11, 14, 15, 16, 17, 18, 20, 23, 25, 26, 27, 28, 29, 30], "DIOsMod2ANr"=[33], "DIOsMod2BNr"=[34], "AIs für \"träge\" Heizungen"=[17, 6, 0, 19, 21, 23], [1, 3, 1, 1], "AnschlüsseHorstMod0"=[enum."1"], "AnschlüsseHorstMod1"=[enum."1", enum."1", enum."1"], "AnschlüsseHorstMod2A"=[enum."1"], "AnschlüsseHorstMod2B"=[enum."1"], "StringSPvorgebenMod0"=[":060A020121"], "StringSPvorgebenMod1"=[":060B020121", ":0618020121", ":060D020121"], "StringSPvorgebenMod2A"=[":0519010104"], "StringSPvorgebenMod2B"=[":060C020121 "], "StringMWAntwort0"=[":060A020121"], "StringMWAntwort1"=[":060B020121", ":0618020121", ":060D020121"], "StringMWAntwort2A"=[":0619020121"], "StringMWAntwort2B"=[":060C020121"], "UmrechnungHorst0"=[0.0003125], "UmrechnungHorst1"=[9.375e-05, 9.375e-05, 9.375e-05], "UmrechnungHorst2A"=[1.0], "UmrechnungHorst2B"=[9.375e-05], "StringMWabfragenMod0"=[":060A0401210120"], "StringMWabfragenMod1"=[":060B0401210120", ":06180401210120", ":060D0401210120"], "StringMWabfragenMod2A"=[":06190401210120"], "StringMWabfragenMod2B"=[":060C0401210120"], "Modul1/AI koeff"=[[-249.333, 111.873, 2.1471], [-249.333, 111.873, 2.1471], [-249.333, 111.873, 2.1471], [-249.333, 111.873, 2.1471], [-237.2852, -153.162, 6.0782], [-237.2852, -153.162, 6.0782], [-249.333, 111.873, 2.1471], [-249.333, 111.873, 2.1471], [-249.333, 111.873, 2.1471], [-249.333, 111.873, 2.1471], [-249.333, 111.873, 2.1471], [-249.333, 111.873, 2.1471], [-249.333, 111.873, 2.1471], [-249.333, 111.873, 2.1471], [-249.333, 111.873, 2.1471], [0.0, 1.0, 0.0], [-249.333, 111.873, 2.1471], [-249.333, 111.873, 2.1471], [-249.333, 111.873, 2.1471], [-249.333, 111.873, 2.1471], [-249.333, 111.873, 2.1471], [-249.333, 111.873, 2.1471], [-249.333, 111.873, 2.1471], [-249.333, 111.873, 2.1471], [0.0, 1.0, 0.0], [0.0, 1.0, 0.0], [0.0, 1.0, 0.0], [0.0, 1.0, 0.0], [0.0, 1.0, 0.0], [0.0, 1.0, 0.0], [0.0, 1.0, 0.0], [0.0, 1.0, 0.0]], "Modul2/AI koeff"=[[0.0, 1.0, 0.0], [0.0, 1.0, 0.0], [0.0, 1.0, 0.0], [0.0, 1.0, 0.0], [0.0, 1.0, 0.0], [0.0, 1.0, 0.0], [0.0, 1.0, 0.0], [0.0, 1.0, 0.0], [0.0, 1.0, 0.0], [0.0, 1.0, 0.0], [0.0, 1.0, 0.0], [0.0, 1.0, 0.0], [0.0, 1.0, 0.0], [0.0, 1.0, 0.0], [0.0, 1.0, 0.0], [0.0, 1.0, 0.0], [0.0, 1.0, 0.0], [0.0, 1.0, 0.0], [0.0, 1.0, 0.0], [0.0, 1.0, 0.0], [0.0, 1.0, 0.0], [0.0, 1.0, 0.0], [0.0, 1.0, 0.0], [0.0, 1.0, 0.0], [0.0, 1.0, 0.0], [0.0, 1.0, 0.0], [0.0, 1.0, 0.0], [0.0, 1.0, 0.0], [0.0, 1.0, 0.0], [0.0, 1.0, 0.0], [0.0, 1.0, 0.0], [0.0, 1.0, 0.0]], "Modul3/AI koeff"=[[0.0, 1.0, 0.0], [0.0, 1.0, 0.0], [0.0, 1.0, 0.0], [0.0, 1.0, 0.0], [0.0, 1.0, 0.0], [0.0, 1.0, 0.0], [0.0, 1.0, 0.0], [0.0, 1.0, 0.0], [0.0, 1.0, 0.0], [0.0, 1.0, 0.0], [0.0, 1.0, 0.0], [0.0, 1.0, 0.0], [0.0, 1.0, 0.0], [0.0, 1.0, 0.0], [0.0, 1.0, 0.0], [0.0, 1.0, 0.0], [0.0, 1.0, 0.0], [0.0, 1.0, 0.0], [0.0, 1.0, 0.0], [0.0, 1.0, 0.0], [0.0, 1.0, 0.0], [0.0, 1.0, 0.0], [0.0, 1.0, 0.0], [0.0, 1.0, 0.0], [0.0, 1.0, 0.0], [0.0, 1.0, 0.0], [0.0, 1.0, 0.0], [0.0, 1.0, 0.0], [0.0, 1.0, 0.0], [0.0, 1.0, 0.0], [0.0, 1.0, 0.0], [0.0, 1.0, 0.0]], "Traps/MachKoeff"=[[0.0, 1.0, 0.0], [-249.333, 111.873, 2.1471], [0.0, 1.0, 0.0], [-249.333, 111.873, 2.1471], [-237.2852, 153.1621, 6.0782], [-237.2852, 153.1621, 6.0782]], "AIsNamen"=["T-MainCol3", "T-Trap1", "T-Trap2", "T-Stirling", "T-PreCol1", "T-PreCol2", "T-MainCol1", "T-MainCol2", "T-T-Line2", "T-MI1", "T-MI2", "T-MI3", "T-MI4", "T-MI5", "T-MI6", "F-MFM1", "T-MainCol4", "T-BHorst1", "T-BHorst2", "T-BHorst3", "T-BHorst4", "T-Oven1", "T-Oven2", "T-T-Line1", "F-MFM2", "P-Me-HP", "P-Me-LP", "P-Vac", "Ref-Turbo", "I-MS-AC", "I-Trap1", "I-Trap2", "Mod2/AI0", "Mod2/AI1", "Mod2/AI2", "Mod2/AI3", "Mod2/AI4", "Mod2/AI5", "Mod2/AI6", "Mod2/AI7", "Mod2/AI8", "Mod2/AI9", "Mod2/AI10", "Mod2/AI11", "Mod2/AI12", "Mod2/AI13", "Mod2/AI14", "Mod2/AI15", "Mod2/AI16", "Mod2/AI17", "Mod2/AI18", "Mod2/AI19", "Mod2/AI20", "Mod2/AI21", "Mod2/AI22", "Mod2/AI23", "Mod2/AI24", "Mod2/AI25", "Mod2/AI26", "Mod2/AI27", "Mod2/AI28", "Mod2/AI29", "Mod2/AI30", "Mod2/AI31", "Mod3/AI0", "Mod3/AI1", "Mod3/AI2", "Mod3/AI3", "Mod3/AI4", "Mod3/AI5", "Mod3/AI6", "Mod3/AI7", "Mod3/AI8", "Mod3/AI9", "Mod3/AI10", "Mod3/AI11", "Mod3/AI12", "Mod3/AI13", "Mod3/AI14", "Mod3/AI15", "Mod3/AI16", "Mod3/AI17", "Mod3/AI18", "Mod3/AI19", "Mod3/AI20", "Mod3/AI21", "Mod3/AI22", "Mod3/AI23", "Mod3/AI24", "Mod3/AI25", "Mod3/AI26", "Mod3/AI27", "Mod3/AI28", "Mod3/AI29", "Mod3/AI30", "Mod3/AI31"], "DIOsMod0Name"=["blindDIO0"], "DIOsMod1Name"=["on/off P-MS", "MS Start", "MS Stop", "FanMach1", "FanReserve", "Valve1A", "on/off PrePump", "Air-In", "on/off VacP2", "on/off VacP1", "S1D", "FanMach2", "S1C", "on/off Stirling", "S1B", "S1A", "Valve1B", "on/off Turbo"], "DIOsMod2AName"=["blindDIO2A"], "DIOsMod2BName"=["blindDIO2B"], "HorstMod0Name"=["MFC1B"], "HorstMod1Name"=["PressContr1A", "PressContr1B", "PressContr1C"], "HorstMod2AName"=["MFC1A"], "HorstMod2BName"=["PressContr1D"], "Startmethode"=0, "Dateiordner Housekeeping"=path "C:/data", "Dateiname Housekeeping"="test"} ("Einstellungen") -> [w110]
    tunnel: [w84] -> w10
    tunnel: "Eingang" -> [w77]
    tunnel: [w73] -> w9
    tunnel: [w55] -> w8
    tunnel: [w53] -> w7
    tunnel: [w52] -> w6
    tunnel: [w42] -> w5
    tunnel: [w37] -> w2
    tunnel: [w36] -> w1
    tunnel: w34 -> [w358]
    tunnel: w33 -> [w420]
    tunnel: w32 -> [w419]
    tunnel: w31 -> [w418]
    tunnel: [w416] -> w30
    tunnel: [w415] -> w29
    tunnel: [w358] -> w28
    tunnel: w27 -> [_]
    tunnel: w26 -> [w356]
    tunnel: w25 -> [w354]
    tunnel: w24 -> [w357]
    tunnel: w23 -> [w355]
    tunnel: w22 -> [w394]
    tunnel: w21 -> [w393]
    tunnel: w20 -> [w392]
    tunnel: w19 -> [w391]
    tunnel: w18 -> [w388]
    tunnel: w17 -> [w384]
    tunnel: w16 -> [w380]
    tunnel: w15 -> [w371]
    tunnel: w14 -> [w377]
    tunnel: w13 -> [w372]
    tunnel: w12 -> [w375]
    tunnel: w11 -> [w374]
    tunnel: "Eingang" -> [w363]
    tunnel: w10 -> [w361]
    tunnel: w9 -> [w352]
    tunnel: w8 -> [w367]
    tunnel: w7 -> [w366]
    tunnel: w6 -> [w365]
    tunnel: w5 -> [w362]
    tunnel: w2 -> [w353]
    tunnel: w1 -> [w350]
    tunnel: w30 -> [w2188]
    tunnel: w29 -> [w2187]
    tunnel: w28 -> [w2186]
    frame #0 {
      w35 = "MFC1A Integriert"
      w79 = string[] ["U_Widr.Trap1 [V]", "Temp.Trap1 [°C]", "U_Widr.Trap2 [V]", "Temp.Trap2 [°C]", "Temp.Mach1 [°C]", "Temp.Mach2 [°C]"]
      w82 = string[] ["Big Ben [s]", "Methodenzeit [s]", "Zykluszeit [s] Mod0", "Zykluszeit [s] Mod1", "Zykluszeit [s] Mod2A", "Zykluszeit [s] Mod2B"]
      w111 = 6  # AnzahlLH
      w38 = FALSE ("Undefinierte Werte möglich")
      w123 = T15 {"Baud Rate"=enum."38.4 kbps", "Data Bits"=enum."8", "Parity"=enum."None", "Stop Bits"=enum."1", "Flow Control"=enum."None"} ("Port-Einstellungen 2")
      w40 = FALSE ("global stop RT")
      w128 = "z"
      w130 = "m"
      w131 = ".tdms" ("String")
      n2 = global write "gvbooleschRT.vi" "global stop RT"(w40) -> ()
      n3 = property on="dargestellte Größe 2" class="Ring (strict)"("AllowUndefVals"=w38) -> ()  [unwired: 2 in, 2 out]
      n4 = property on="Zeitachse2" class="Ring (strict)"("AllowUndefVals"=w38) -> ()  [unwired: 2 in, 2 out]
      n5 = property on="Zeitachse1" class="Ring (strict)"("AllowUndefVals"=w38) -> ()  [unwired: 2 in, 2 out]
      n6 = property on="dargestellte Größe 1" class="Ring (strict)"("AllowUndefVals"=w38) -> ()  [unwired: 2 in, 2 out]
      n7 = property on="Methodennummer" class="Ring (strict)"("AllowUndefVals"=w38) -> ()  [unwired: 2 in, 2 out]
      n8 = Array Size(array=w77) -> (size(s)=w76:i32)
      n9 = for {
        N: w76 -> [_]
        tunnel: [w174] -> w75 mode=indexing
        i -> [w175]
        n10 = Number To Decimal String(number=w175) -> (decimal integer string=w174:string)  [unwired: 1 in]
      }
      n11 = case shown="True" "Dateien fürs MS schicken?" {
        tunnel: [path "" ("path") w160] -> w55
        frame False {
        }
        frame True {
          n12 = Open/Create/Replace File(file path (use dialog)="Pfad MS-Datei CRIO", operation (0:open)=T6."replace or create" ("Operation (0:Öffnen)")) -> (refnum out=w169:refnum<file>, error out=w168:errorcluster)  [unwired: 4 in, 1 out]
          n13 = Open/Create/Replace File(file path (use dialog)=path "c:/fromcriordy.txt" ("Dateipfad (Dialog verwenden)"), operation (0:open)=T6."replace or create" ("Operation (0:Öffnen)")) -> (refnum out=w163:refnum<file>, error out=w164:errorcluster)  [unwired: 4 in, 1 out]
          n14 = Write to Text File(file (use dialog)=w169, text="Text0 MS-Datei", error in=w168) -> (refnum out=w166:refnum<file>, error out=w165:errorcluster)  [unwired: 1 in, 1 out]
          n15 = Close File(refnum=w163, error in=w164) -> (path=w160:path)  [unwired: 1 out]
          n16 = Close File(refnum=w166, error in=w165) -> ()  [unwired: 2 out]
        }
      }
      n17 = local write "global stop RT"(w40) -> ()
      n18 = xnode "Open FPGA VI Reference"() -> ("FPGA VI Reference Out"=w157:refnum<k20>, "error out"=w158:errorcluster)  [unwired: 2 in]
      n19 = xnode "Invoke Method"("FPGA VI Reference In"=w157, "error in"=w158) -> ("FPGA VI Reference Out"=w156:refnum<k20>, "error out"=w155:errorcluster)
      n20 = property on="Methodennummer" class="Ring (strict)"("Strings []"=w75) -> ()  [unwired: 2 in, 2 out]
      n21 = Number To Decimal String(number=0 ("Wert")) -> (decimal integer string=w132:string)  [unwired: 1 in]
      n22 = Number To Decimal String(number=1 ("Wert")) -> (decimal integer string=w127:string)  [unwired: 1 in]
      n23 = xnode "Read/Write Control"("FPGA VI Reference In"=w156, "error in"=w155, "vor der Messung [us]Mach"=u16 600 ("vor der Messung [us]Mach1"), "wie viele Messwerte?Mach"=u16 14 ("wie viele Messwerte?Mach1"), "Abstand zwischen Messungen [us]Mach"=u16 150 ("Abstand zwischen Messungen [us]Mach1"), "Heizen?Trap1"=FALSE, "Heizen?Trap2"=FALSE, "warten[us]Trap1"=u32 2000, "warten[us]Trap2"=u32 2000, "Per[us]Trap1"=u32 10000, "Per[us]Trap2"=u32 10000, "global stop"=FALSE, "Per[us]Mach"=u16 20000 ("Per[us]Mach1"), "Heizen?Mach1"=FALSE, "Heizen?Mach2"=FALSE, "Port 1"=w123, "Port 2"=w123, "Port 3"=w123, "Port 4"=w123, "Port 5"=w123, "Port 6"=w123, "Port 7"=w123, "Port 8"=w123, "ServosPeriode(us)"=u32 20000, "Servo1WarmHigh(us)"=u32 1430, "Servo1KaltHigh(us)"=u32 1630, "Servo2WarmHigh(us)"=u32 1320, "Servo2KaltHigh(us)"=u32 1520) -> ("FPGA VI Reference Out"=w154:refnum<k20>, "error out"=w153:errorcluster)
      n24 = xnode "Invoke Method"("FPGA VI Reference In"=w154, "error in"=w153) -> ("FPGA VI Reference Out"=w122:refnum<k20>, "error out"=w115:errorcluster)  [unwired: 1 in]
      n25 = Unbundle(w110) -> ("DIOsMod0Nr"=w72:i32[], "DIOsMod1Nr"=w71:i32[], "DIOsMod2ANr"=w70:i32[], "DIOsMod2BNr"=w69:i32[], "AIs für \"träge\" Heizungen"=w109:i32[], w108:i32[], "AnschlüsseHorstMod0"=w67:T16, "AnschlüsseHorstMod1"=w66:T16, "AnschlüsseHorstMod2A"=w65:T16, "AnschlüsseHorstMod2B"=w64:T16, "StringSPvorgebenMod0"=w107:string[], "StringSPvorgebenMod1"=w106:string[], "StringSPvorgebenMod2A"=w105:string[], "StringSPvorgebenMod2B"=w104:string[], "StringMWAntwort0"=w102:string[], "StringMWAntwort1"=w101:string[], "StringMWAntwort2A"=w100:string[], "StringMWAntwort2B"=w99:string[], "UmrechnungHorst0"=w98:dbl[], "UmrechnungHorst1"=w97:dbl[], "UmrechnungHorst2A"=w96:dbl[], "UmrechnungHorst2B"=w95:dbl[], "StringMWabfragenMod0"=w93:string[], "StringMWabfragenMod1"=w92:string[], "StringMWabfragenMod2A"=w91:string[], "StringMWabfragenMod2B"=w90:string[], "Modul1/AI koeff"=w88:dbl[][], "Modul2/AI koeff"=w87:dbl[][], "Modul3/AI koeff"=w86:dbl[][], "Traps/MachKoeff"=w85:dbl[][], "AIsNamen"=w80:string[], "DIOsMod0Name"=w51:string[], "DIOsMod1Name"=w50:string[], "DIOsMod2AName"=w49:string[], "DIOsMod2BName"=w48:string[], "HorstMod0Name"=w47:string[], "HorstMod1Name"=w46:string[], "HorstMod2AName"=w45:string[], "HorstMod2BName"=w44:string[], "Startmethode"=w54:i32, "Dateiordner Housekeeping"=w52:path, "Dateiname Housekeeping"=w53:string)
      n26 = property on="Methodennummer" class="Ring (strict)"("Value"=w54) -> ()  [unwired: 2 in, 2 out]
      n27 = Number To Decimal String(number=w54) -> (decimal integer string=w129:string)  [unwired: 1 in]
      n28 = Concatenate Strings(w53, w130, w129, w128, w132, w131) -> (w136:string)
      n29 = Concatenate Strings(w53, w130, w129, w128, w127, w131) -> (w135:string)
      n30 = Build Path(base path=w52, name or relative path=w136) -> (appended path=w137:path)
      n31 = Build Path(base path=w52, name or relative path=w135) -> (appended path=w126:path)
      n32 = Build Array (concatenate)(w67, w66, w65, w64) -> (w63:T16)
      n33 = Build Array (concatenate)(w47, w46, w45, w44) -> (w78:string[])
      n34 = Build Array (concatenate)(w107, w106, w105, w104) -> (w103:string[])
      n35 = TDMS Open(10:T5."create" ("Operation (0:Öffnen)"), 11:w137) -> (3:w124:refnum<k34>)  [unwired: 4 in, 1 out]
      n36 = xnode "Read/Write Control"("FPGA VI Reference In"=w122, "error in"=w115, "Update Config"=TRUE) -> ("FPGA VI Reference Out"=w117:refnum<k20>, "error out"=w114:errorcluster)
      n37 = Build Array (concatenate)(w93, w92, w91, w90) -> (w89:string[])
      n38 = Build Array (concatenate)(w102, w101, w100, w99) -> (w94:string[])
      n39 = local write "aktuelle TDMS-Datei"(w124) -> ()
      n40 = Add Array Elements(numeric array=w108) -> (sum=w36:i32)
      n41 = Build Array (concatenate)(w98, w97, w96, w95) -> (w74:dbl[])
      n42 = xnode "Invoke Method"("FPGA VI Reference In"=w117, "error in"=w114, "Number of Elements"=u32 0) -> ("FPGA VI Reference Out"=w116:refnum<k20>, "error out"=w120:errorcluster, "Elements Remaining"=w118:u32)  [unwired: 1 in, 1 out]
      n43 = Split 1D Array(array=w82, index=2 ("Index")) -> (second subarray=w41:string[])  [unwired: 1 out]
      n44 = property on="Zeitachse1" class="Ring (strict)"("Strings []"=w41) -> ()  [unwired: 2 in, 2 out]
      n45 = property on="Zeitachse2" class="Ring (strict)"("Strings []"=w41) -> ()  [unwired: 2 in, 2 out]
      n46 = Build Array (concatenate)(w80, w79, w78, w35) -> (w39:string[])
      n47 = Build Cluster Array(w72, w71, w70, w69) -> (w68:cluster{"DIOsMod2BNr":i32[]}[])
      n48 = for {
        tunnel: w68 -> [w177] mode=indexing
        tunnel: [w178] -> w62 mode=indexing
        n49 = Unbundle(w177) -> ("DIOsMod2BNr"=w176:i32[])
        n50 = Array Size(array=w176) -> (size(s)=w178:i32)
      }
      n51 = property on="dargestellte Größe 1" class="Ring (strict)"("Strings []"=w39) -> ()  [unwired: 2 in, 2 out]
      n52 = property on="dargestellte Größe 2" class="Ring (strict)"("Strings []"=w39) -> ()  [unwired: 2 in, 2 out]
      n53 = xnode "Invoke Method"("FPGA VI Reference In"=w116, "error in"=w120, "Number of Elements"=w118) -> ("FPGA VI Reference Out"=w113:refnum<k20>, "error out"=w112:errorcluster)  [unwired: 1 in, 2 out]
      n54 = Bundle("DIOsMod0Name"=w51, "DIOsMod1Name"=w50, "DIOsMod2AName"=w49, "DIOsMod2BName"=w48, "HorstMod0Name"=w47, "HorstMod1Name"=w46, "HorstMod2AName"=w45, "HorstMod2BName"=w44, string[] ["Horst1", "MainCol1", "MainCol2", "Horst2", "Oven", "T-Line"]) -> (w42:T17)  [unwired: 1 in]
      n55 = TDMS Open(10:T5."create" ("Operation (0:Öffnen)"), 11:w126) -> (3:w125:refnum<k34>)  [unwired: 4 in, 1 out]
      n56 = Build Array (concatenate)(string[] ["Datei Nr.", "Zyklusnr. Mod0", "Zyklusnr. Mod1", "Zyklusnr. Mod2A", "Zyklusnr. Mod2B"], w82, w80, w79, w78, w35) -> (w84:string[])
      n57 = for {
        N: w36 -> [_]
        tunnel: [0.0] -> w73 mode=indexing
        tunnel: ["nix"] -> w37 mode=indexing
      }
    }
    frame #1 {
      w364 = dbl[] []
      n58 = while "\"langsame\" Regelungen" {
        tunnel: w388 -> [w1002]
        stop <- w1012 stop-if-true
        w1010 = cluster{"output high":dbl, "output low":dbl} {"output high"=100.0, "output low"=0.0} ("output range")
        n59 = local read "Mod1/AI"() -> (w1003:dbl[])
        n60 = local read "PIDs für \"träge\" Heizungen"() -> (w977:T3)
        n61 = call "Warten29"("Count(mSec)"=u32 100) -> ()  [unwired: 1 out]
        n62 = for {
          tunnel: w1003 -> [w1015]
          tunnel: w1002 -> [w1014] mode=indexing
          tunnel: [w1013] -> w1001 mode=indexing
          n63 = Index Array(array=w1015, index=w1014) -> (element=w1013:dbl)
        }
        n64 = Array To Cluster(array=w977) -> (cluster=w976:T18)
        n65 = Array To Cluster(array="LangsameHeizungenSP") -> (cluster=w992:T19)
        n66 = Array To Cluster(array=w1001) -> (cluster=w1000:T20)
        n67 = Unbundle "Horst1\nMainCol1\nMainCol2\nHorst2\nOven\nT-line"(w992) -> ("LangsameHeizungenSP[0]"=w991:dbl, "LangsameHeizungenSP[1]"=w990:dbl, "LangsameHeizungenSP[2]"=w989:dbl, "LangsameHeizungenSP[3]"=w988:dbl, "LangsameHeizungenSP[4]"=w987:dbl, "LangsameHeizungenSP[5]"=w986:dbl)
        n68 = Unbundle "Horst1\nMainCol1\nMainCol2\nHorst2\nOven\nT-Line"(w1000) -> ("[0]"=w999:dbl, "[1]"=w998:dbl, "[2]"=w997:dbl, "[3]"=w996:dbl, "[4]"=w995:dbl, "[5]"=w994:dbl)
        n69 = Unbundle "Horst1\nMainCol1\nMainCol2\nHorst2\nOven\nT-Line"(w976) -> ("PIDs für \"träge\" Heizungen[0]"=w1009:T21, "PIDs für \"träge\" Heizungen[1]"=w1008:T21, "PIDs für \"träge\" Heizungen[2]"=w1007:T21, "PIDs für \"träge\" Heizungen[3]"=w1006:T21, "PIDs für \"träge\" Heizungen[4]"=w1005:T21, "PIDs für \"träge\" Heizungen[5]"=w1004:T21)
        n70 = call-poly <vilib>:"PID.vi"("output range"=w1010, "PID gains"=w1008, "process variable"=w998, "setpoint"=w990) -> ("output"=w984:dbl)  [unwired: 6 in, 1 out]
        n71 = call-poly <vilib>:"PID.vi"("output range"=w1010, "PID gains"=w1007, "process variable"=w997, "setpoint"=w989) -> ("output"=w983:dbl)  [unwired: 6 in, 1 out]
        n72 = call-poly <vilib>:"PID.vi"("output range"=w1010, "PID gains"=w1009, "process variable"=w999, "setpoint"=w991) -> ("output"=w985:dbl)  [unwired: 6 in, 1 out]
        n73 = call-poly <vilib>:"PID.vi"("output range"=w1010, "PID gains"=w1006, "process variable"=w996, "setpoint"=w988) -> ("output"=w982:dbl)  [unwired: 6 in, 1 out]
        n74 = call-poly <vilib>:"PID.vi"("output range"=w1010, "PID gains"=w1004, "process variable"=w994, "setpoint"=w986) -> ("output"=w980:dbl)  [unwired: 6 in, 1 out]
        n75 = call-poly <vilib>:"PID.vi"("output range"=w1010, "PID gains"=w1005, "process variable"=w995, "setpoint"=w987) -> ("output"=w981:dbl)  [unwired: 6 in, 1 out]
        n76 = Build Array(w985, w984, w983, w982, w981, w980) -> (w979:dbl[])
        n77 = To Unsigned Long Integer(number=w979) -> (unsigned 32bit integer=w978:u32[])
        n78 = local write "LangsameHeizungen%"(w978) -> ()
        n79 = global read "gvbooleschRT.vi" "global stop RT"() -> (w1012:bool)
      }
      n80 = while {
        shift-right: ["Methodennummer"] -> _
        shift-left: w420 -> [w2179]
        stop <- w2181 stop-if-true
        n81 = call "Warten"("Count(mSec)"=u32 1000) -> ()  [unwired: 1 out]
        n82 = Not Equal?(x=w2179, y="Methodennummer") -> (x != y?=→"Methodenwechsel?":bool)
        n83 = global read "gvbooleschRT.vi" "global stop RT"() -> (w2181:bool)
      }
      n84 = while "\"langsame\" Pulse" {
        tunnel: w358 -> [w789]
        stop <- w790 stop-if-true
        n85 = Array To Cluster(array="Heizen?LH") -> (cluster=w760:T22)
        n86 = Unbundle(w760) -> ("Heizen?LH[0]"=w759:bool, "Heizen?LH[1]"=w758:bool, "Heizen?LH[2]"=w757:bool, "Heizen?LH[3]"=w756:bool, "Heizen?LH[4]"=w755:bool, "Heizen?LH[5]"=w754:bool)
        n87 = xnode "Read/Write Control"("FPGA VI Reference In"=w789, "on/off Bronkhorst I Heater"=w759, "on/off Main-Col I Heater"=w758, "on/off Main-Col II Heater"=w757, "on/off Bronkhorst II Heater"=w756, "on/off Oven Heater"=w755, "on/off T-Line Heater"=w754) -> ("FPGA VI Reference Out"=w770:refnum<k20>)  [unwired: 1 in, 1 out]
        n88 = Array To Cluster(array="LangsameHeizungen%") -> (cluster=w768:T23)
        n89 = Unbundle "Horst1\nMainCol1\nMainCol2\nHorst2\nOven\nT-Line"(w768) -> ("LangsameHeizungen%[0]"=w767:u32, "LangsameHeizungen%[1]"=w766:u32, "LangsameHeizungen%[2]"=w765:u32, "LangsameHeizungen%[3]"=w764:u32, "LangsameHeizungen%[4]"=w763:u32, "LangsameHeizungen%[5]"=w762:u32)
        n90 = for {
          N: 1 -> [_]
          tunnel: w770 -> [w860]
          tunnel: [w860] -> w778
          tunnel: w767 -> [w859]
          n91 = call "Warten21"("Count(mSec)"=w859) -> ()  [unwired: 1 out]
        }
        n92 = for {
          N: 1 -> [_]
          tunnel: w770 -> [w837]
          tunnel: [w837] -> w775
          tunnel: w766 -> [w836]
          n93 = call "Warten24"("Count(mSec)"=w836) -> ()  [unwired: 1 out]
        }
        n94 = for {
          N: 1 -> [_]
          tunnel: w770 -> [w814]
          tunnel: [w814] -> w772
          tunnel: w765 -> [w813]
          n95 = call "Warten30"("Count(mSec)"=w813) -> ()  [unwired: 1 out]
        }
        n96 = for {
          N: 1 -> [_]
          tunnel: w770 -> [w906]
          tunnel: [w906] -> w784
          tunnel: w764 -> [w905]
          n97 = call "Warten15"("Count(mSec)"=w905) -> ()  [unwired: 1 out]
        }
        n98 = for {
          N: 1 -> [_]
          tunnel: w770 -> [w883]
          tunnel: [w883] -> w781
          tunnel: w763 -> [w882]
          n99 = call "Warten18"("Count(mSec)"=w882) -> ()  [unwired: 1 out]
        }
        n100 = for {
          N: 1 -> [_]
          tunnel: w770 -> [w929]
          tunnel: [w929] -> w787
          tunnel: w762 -> [w928]
          n101 = call "Warten12"("Count(mSec)"=w928) -> ()  [unwired: 1 out]
        }
        n102 = call "Warten9"("Count(mSec)"=u32 100) -> ()  [unwired: 1 out]
        n103 = xnode "Read/Write Control"("FPGA VI Reference In"=w778, "on/off Bronkhorst I Heater"=FALSE ("on/off T-Line Heater")) -> ()  [unwired: 1 in, 2 out]
        n104 = xnode "Read/Write Control"("FPGA VI Reference In"=w775, "on/off Main-Col I Heater"=FALSE ("on/off T-Line Heater")) -> ()  [unwired: 1 in, 2 out]
        n105 = xnode "Read/Write Control"("FPGA VI Reference In"=w772, "on/off Main-Col II Heater"=FALSE ("on/off T-Line Heater")) -> ()  [unwired: 1 in, 2 out]
        n106 = xnode "Read/Write Control"("FPGA VI Reference In"=w784, "on/off Bronkhorst II Heater"=FALSE ("on/off T-Line Heater")) -> ()  [unwired: 1 in, 2 out]
        n107 = xnode "Read/Write Control"("FPGA VI Reference In"=w781, "on/off Oven Heater"=FALSE ("on/off T-Line Heater")) -> ()  [unwired: 1 in, 2 out]
        n108 = xnode "Read/Write Control"("FPGA VI Reference In"=w787, "on/off T-Line Heater"=FALSE) -> ()  [unwired: 1 in, 2 out]
        n109 = global read "gvbooleschRT.vi" "global stop RT"() -> (w790:bool)
      }
      n110 = while {
        shift-right: [w1338] -> _
        shift-left: w364 -> [w1332]
        shift-right: [w1337] -> _
        shift-left: w364 -> [w1330]
        shift-right: [w1335] -> _
        shift-left: w364 -> [w1336]
        shift-right: [w1333] -> _
        shift-left: w364 -> [w1334]
        shift-right: [w1339] -> _
        shift-left: _ -> [w1340]
        shift-right: ["dargestellte Größe 1"] -> _
        shift-left: _ -> [w1322]
        shift-right: ["Zeitachse1"] -> _
        shift-left: _ -> [w1324]
        shift-right: [w1312] -> _
        shift-left: w364 -> [w1320]
        shift-right: [w1313] -> _
        shift-left: w364 -> [w1319]
        shift-right: [w1318] -> _
        shift-left: w364 -> [w1316]
        shift-right: [w1317] -> _
        shift-left: w364 -> [w1315]
        shift-right: [w1305] -> _
        shift-left: _ -> [w1306]
        shift-right: ["Zeitachse2"] -> _
        shift-left: _ -> [w1304]
        shift-right: ["dargestellte Größe 2"] -> _
        shift-left: _ -> [w1303]
        stop <- w1343 stop-if-true
        w1287 = 0.0 ("X-Achse.Bereich:Minimum")
        n111 = local read "Big Ben, Methodenzeit, Zykluszeit0, Zykluszeit1, Zykluszeit2A, Zykluszeit2B"() -> (w1311:dbl[])
        n112 = local read "Zykluslängen [s]"() -> (w1286:dbl[])
        n113 = local read "Zyklusnummern 0, 1, 2A, 2B"() -> (w1307:i32[])
        n114 = property on="Anzeige2" class="XYGraph (strict)"("XScale.Minimum"=w1287) -> ()  [unwired: 2 in, 2 out]
        n115 = property on="Anzeige1" class="XYGraph (strict)"("XScale.Minimum"=w1287) -> ()  [unwired: 2 in, 2 out]
        n116 = Index Array(array=w1286, index="Zeitachse2") -> (element=w1280:dbl)
        n117 = property on="Anzeige2" class="XYGraph (strict)"("XScale.Maximum"=w1280) -> ()  [unwired: 2 in, 2 out]
        n118 = Divide(x=w1280, y=20.0) -> (x/y=w1281:dbl)
        n119 = property on="Anzeige2" class="XYGraph (strict)"("XScale.Increment"=w1281) -> ()  [unwired: 2 in, 2 out]
        n120 = local read "Traps/Machs"() -> (w1294:dbl[])
        n121 = local read "veränderte Methode benutzen"() -> (w1276:bool)
        n122 = local read "Mod2/AI"() -> (w1296:dbl[])
        n123 = Index Array(array=w1307, index="Zeitachse1") -> (element=w1339:i32)
        n124 = local read "MFC1A Integriert"() -> (w1268:dbl)
        n125 = local read "Methodenwechsel?"() -> (w1275:bool)
        n126 = local read "MWHorst"() -> (w1321:dbl[])
        n127 = local read "Mod3/AI"() -> (w1295:dbl[])
        n128 = local read "Mod1/AI"() -> (w1297:dbl[])
        n129 = Add(x="Zeitachse2", y=2) -> (x+y=w1288:i32)
        n130 = Index Array(array=w1307, index="Zeitachse2") -> (element=w1305:i32)
        n131 = Not Equal?(x=w1340, y=w1339) -> (x != y?=w1328:bool)
        n132 = Not Equal?(x="Zeitachse1", y=w1324) -> (x != y?=w1326:bool)
        n133 = Not Equal?(x=w1306, y=w1305) -> (x != y?=w1301:bool)
        n134 = Not Equal?(x=w1304, y="Zeitachse2") -> (x != y?=w1300:bool)
        n135 = Not Equal?(x=w1303, y="dargestellte Größe 2") -> (x != y?=w1298:bool)
        n136 = Or(x=w1301, y=w1300) -> (x .or. y?=w1299:bool)
        n137 = Or(x=w1299, y=w1298) -> (x .or. y?=w1292:bool)
        n138 = Not Equal?(x="dargestellte Größe 1", y=w1322) -> (x != y?=w1325:bool)
        n139 = Or(x=w1328, y=w1326) -> (x .or. y?=w1327:bool)
        n140 = Build Array (concatenate)(w1297, w1296, w1295, w1294, w1321, w1268) -> (w1310:dbl[])
        n141 = Add(x="Zeitachse1", y=2) -> (x+y=w1285:i32)
        n142 = Or(x=w1275, y=w1276) -> (x .or. y?=w1271:bool)
        n143 = Index Array(array=w1311, index=w1288) -> (element=w1308:dbl)
        n144 = Index Array(array=w1310, index="dargestellte Größe 2") -> (element=w1309:dbl)
        n145 = Or(x=w1327, y=w1325) -> (x .or. y?=w1291:bool)
        n146 = Index Array(array=w1311, index=w1285) -> (element=w1331:dbl)
        n147 = Index Array(array=w1310, index="dargestellte Größe 1") -> (element=w1329:dbl)
        n148 = Or(x="Tafel putzen2", y=w1292) -> (x .or. y?=w1273:bool)
        n149 = Or(x=w1273, y=w1271) -> (x .or. y?=w1272:bool)
        n150 = Or(x="Tafel putzen1", y=w1291) -> (x .or. y?=w1270:bool)
        n151 = Or(x=w1271, y=w1270) -> (x .or. y?=w1269:bool)
        n152 = case shown="True" w1269 {
          tunnel: w1332 -> [w1364 w1368]
          tunnel: [w1362 w1372] -> w1338
          tunnel: [w1359 w1369] -> w1337
          tunnel: w1336 -> [w1366 _]
          tunnel: [w1366 w1368] -> w1335
          tunnel: w1334 -> [w1365 _]
          tunnel: [w1365 w1367] -> w1333
          tunnel: w1331 -> [w1363 w1373]
          tunnel: w1330 -> [w1361 w1367]
          tunnel: w1329 -> [w1360 w1370]
          frame False {
            n153 = Build Array (concatenate)(w1364, w1363) -> (w1362:dbl[])
            n154 = Build Array (concatenate)(w1361, w1360) -> (w1359:dbl[])
          }
          frame True {
            w1371 = dbl[] []
            n155 = Build Array (concatenate)(w1371, w1373) -> (w1372:dbl[])
            n156 = Build Array (concatenate)(w1371, w1370) -> (w1369:dbl[])
          }
        }
        n157 = case shown="True" w1272 {
          tunnel: w1320 -> [w1349 w1353]
          tunnel: [w1347 w1357] -> w1312
          tunnel: [w1344 w1354] -> w1313
          tunnel: w1316 -> [w1351 _]
          tunnel: [w1351 w1353] -> w1318
          tunnel: w1315 -> [w1350 _]
          tunnel: [w1350 w1352] -> w1317
          tunnel: w1308 -> [w1348 w1358]
          tunnel: w1319 -> [w1346 w1352]
          tunnel: w1309 -> [w1345 w1355]
          frame False {
            n158 = Build Array (concatenate)(w1349, w1348) -> (w1347:dbl[])
            n159 = Build Array (concatenate)(w1346, w1345) -> (w1344:dbl[])
          }
          frame True {
            w1356 = dbl[] []
            n160 = Build Array (concatenate)(w1356, w1358) -> (w1357:dbl[])
            n161 = Build Array (concatenate)(w1356, w1355) -> (w1354:dbl[])
          }
        }
        n162 = call "Warten6"("Count(mSec)"=u32 100) -> ()  [unwired: 1 out]
        n163 = Index Array(array=w1286, index="Zeitachse1") -> (element=w1284:dbl)
        n164 = Divide(x=w1284, y=20.0) -> (x/y=w1282:dbl)
        n165 = property on="Anzeige1" class="XYGraph (strict)"("XScale.Maximum"=w1284) -> ()  [unwired: 2 in, 2 out]
        n166 = property on="Anzeige1" class="XYGraph (strict)"("XScale.Increment"=w1282) -> ()  [unwired: 2 in, 2 out]
        n167 = global read "gvbooleschRT.vi" "global stop RT"() -> (w1343:bool)
        n168 = Bundle(w1338, w1337) -> (→"Anzeige1":cluster{dbl[], dbl[]})  [unwired: 1 in]
        n169 = Bundle(w1312, w1313) -> (→"Anzeige2":cluster{dbl[], dbl[]})  [unwired: 1 in]
      }
      n170 = while {
        tunnel: w363 -> [w596]
        tunnel: w362 -> [w593]
        stop <- w597 stop-if-true
        n171 = local read "Methodennummer"() -> (w595:i32)
        n172 = Index Array(array=w596, index=w595) -> (element=w594:T2)
        n173 = while {
          shift-right: [w599] -> _
          shift-left: w594 -> [w600]
          tunnel: w593 -> [w598]
          stop <- w603 stop-if-true
          n174 = call "Warten19"("Count(mSec)"=u32 500) -> ()  [unwired: 1 out]
          n175 = case shown="True" "Methode verändern" {
            tunnel: w600 -> [w606 w610]
            tunnel: [w606 w609] -> w599
            tunnel: w598 -> [_ w607]
            frame False {
            }
            frame True {
              n176 = call "methodeändern.vi"("Methode"=w610, "Namen"=w607) -> ("Methode"=w609:T24)  [unwired: 1 in]
              "Ausgang" <- w609
              n177 = property on="Methode verändern" class="Bool (strict)"("Value"=FALSE ("Methode verändern")) -> ()  [unwired: 2 in, 2 out]
            }
          }
          "veränderte Methode" <- w599
          n178 = local read "Methodenwechsel?"() -> (w605:bool)
          n179 = global read "gvbooleschRT.vi" "global stop RT"() -> (w604:bool)
          n180 = Or(x=w605, y=w604) -> (x .or. y?=w603:bool)
        }
        n181 = global read "gvbooleschRT.vi" "global stop RT"() -> (w597:bool)
      }
      n182 = Add Array Elements(numeric array=w371) -> (sum=w370:i32)
      n183 = Compound Arithmetic op=ADD(w370, 8 ("Wert"), w372, w377) -> (w376:i32)
      n184 = for {
        N: w376 -> [_]
        tunnel: [FALSE] -> w379 mode=indexing
        tunnel: [0.0] -> w373 mode=indexing
      }
      n185 = Index Array(array=w393, index (col)=2 ("Deaktivierter Index (Spalte)")) -> (element=w411:dbl[])  [unwired: 1 in]
      n186 = Index Array(array=w393, index (col)=1 ("Deaktivierter Index (Spalte)")) -> (element=w409:dbl[])  [unwired: 1 in]
      n187 = Index Array(array=w393, index (col)=0 ("Deaktivierter Index (Spalte)")) -> (element=w407:dbl[])  [unwired: 1 in]
      n188 = Index Array(array=w392, index (col)=2 ("Deaktivierter Index (Spalte)")) -> (element=w403:dbl[])  [unwired: 1 in]
      n189 = Index Array(array=w392, index (col)=1 ("Deaktivierter Index (Spalte)")) -> (element=w402:dbl[])  [unwired: 1 in]
      n190 = Index Array(array=w392, index (col)=0 ("Deaktivierter Index (Spalte)")) -> (element=w401:dbl[])  [unwired: 1 in]
      n191 = Index Array(array=w391, index (col)=2 ("Deaktivierter Index (Spalte)")) -> (element=w397:dbl[])  [unwired: 1 in]
      n192 = Index Array(array=w391, index (col)=1 ("Deaktivierter Index (Spalte)")) -> (element=w396:dbl[])  [unwired: 1 in]
      n193 = Index Array(array=w391, index (col)=0 ("Deaktivierter Index (Spalte)")) -> (element=w395:dbl[])  [unwired: 1 in]
      n194 = Index Array(array=w384, index (col)=2 ("Deaktivierter Index (Spalte)")) -> (element=w383:dbl[])  [unwired: 1 in]
      n195 = Index Array(array=w384, index (col)=1 ("Deaktivierter Index (Spalte)")) -> (element=w382:dbl[])  [unwired: 1 in]
      n196 = Index Array(array=w384, index (col)=0 ("Deaktivierter Index (Spalte)")) -> (element=w381:dbl[])  [unwired: 1 in]
      n197 = while {
        stop <- w1032 stop-if-true
        w1017 = 10.0
        n198 = call "Warten27"("Count(mSec)"=u32 1000) -> ()  [unwired: 1 out]
        n199 = local read "Traps/Machs"() -> (w1019:dbl[])
        n200 = local read "Mod1/AI"() -> (w1030:dbl[])
        n201 = local read "Mod2/AI"() -> (w1029:dbl[])
        n202 = local read "Mod3/AI"() -> (w1028:dbl[])
        n203 = for {
          N: 9 -> [_]
          shift-right: [w1039] -> w1026
          shift-left: w1030 -> [w1040]
          shift-right: [w1037] -> w1025
          shift-left: w1029 -> [w1038]
          shift-right: [w1035] -> w1024
          shift-left: w1028 -> [w1036]
          shift-right: [w1033] -> w1018
          shift-left: w1019 -> [w1034]
          n204 = flat-sequence {
            tunnel: w1040 -> [w1053]
            tunnel: [w1051] -> w1039
            tunnel: w1038 -> [w1050]
            tunnel: [w1048] -> w1037
            tunnel: w1036 -> [w1047]
            tunnel: [w1045] -> w1035
            tunnel: w1034 -> [w1043]
            tunnel: [w1042] -> w1033
            frame #0 {
              n205 = call "Warten28"("Count(mSec)"=u32 100) -> ()  [unwired: 1 out]
            }
            frame #1 {
              n206 = local read "Traps/Machs"() -> (w1044:dbl[])
              n207 = local read "Mod1/AI"() -> (w1052:dbl[])
              n208 = local read "Mod2/AI"() -> (w1049:dbl[])
              n209 = local read "Mod3/AI"() -> (w1046:dbl[])
              n210 = Add(x=w1053, y=w1052) -> (x+y=w1051:dbl[])
              n211 = Add(x=w1050, y=w1049) -> (x+y=w1048:dbl[])
              n212 = Add(x=w1047, y=w1046) -> (x+y=w1045:dbl[])
              n213 = Add(x=w1044, y=w1043) -> (x+y=w1042:dbl[])
            }
          }
        }
        n214 = Divide(x=w1026, y=w1017) -> (x/y=w1023:dbl[])
        n215 = Divide(x=w1025, y=w1017) -> (x/y=w1022:dbl[])
        n216 = Divide(x=w1024, y=w1017) -> (x/y=w1021:dbl[])
        n217 = Divide(x=w1018, y=w1017) -> (x/y=w1016:dbl[])
        n218 = Build Array (concatenate)(w1023, w1022, w1021, w1016) -> (→"Mod1Mod2Mod3/AITrapsMachs1Hz":dbl[])
        n219 = global read "gvbooleschRT.vi" "global stop RT"() -> (w1032:bool)
      }
      n220 = for {
        N: 64 -> [_]
        tunnel: [FALSE] -> w389 mode=indexing
      }
      n221 = while {
        tunnel: w379 -> [w1413]
        tunnel: w371 -> [w1392]
        tunnel: w377 -> [w1397]
        tunnel: w372 -> [w1399]
        tunnel: w374 -> [w1409]
        tunnel: w373 -> [w1407]
        tunnel: w370 -> [w1391]
        stop <- "global stop RT" stop-if-true
        w1385 = 2 ("Index")
        w1404 = 6 ("Index")
        n222 = local read "Zwangsbedingungen"() -> (w1395:dbl[][])
        n223 = local read "Mod1Mod2Mod3/AITrapsMachs1Hz"() -> (w1416:dbl[])
        n224 = call "Warten5"("Count(mSec)"=u32 1000) -> ()  [unwired: 1 out]
        n225 = local read "MWHorst"() -> (w1415:dbl[])
        n226 = Build Array (concatenate)(w1416, w1415) -> (w1414:dbl[])
        n227 = for {
          tunnel: w1414 -> [w1452]
          tunnel: w1395 -> [w1456] mode=indexing
          shift-right: [w1460] -> w1412
          shift-left: w1413 -> [w1465]
          shift-right: [w1461] -> w1406
          shift-left: w1407 -> [w1464]
          n228 = Index Array(array=w1456, index=0 ("Index")) -> (element=w1476:dbl)
          n229 = Index Array(array=w1456, index=3 ("Index")) -> (element=w1451:dbl)
          n230 = Index Array(array=w1456, index=1 ("Index")) -> (element=w1474:dbl)
          n231 = Index Array(array=w1456, index=4 ("Index")) -> (element=w1450:dbl)
          n232 = Index Array(array=w1456, index=2 ("Index")) -> (element=w1470:dbl)
          n233 = Index Array(array=w1456, index=5 ("Index")) -> (element=w1449:dbl)
          n234 = Index Array(array=w1456, index=6 ("Index")) -> (element=w1467:dbl)
          n235 = Index Array(array=w1456, index=7 ("Index")) -> (element=w1462:dbl)
          n236 = To Long Integer(number=w1476) -> (32bit integer=w1469:i32)
          n237 = To Long Integer(number=w1474) -> (32bit integer=w1473:i32)
          n238 = To Long Integer(number=w1467) -> (32bit integer=w1463:i32)
          n239 = To Long Integer(number=w1451) -> (32bit integer=w1453:i32)
          n240 = To Long Integer(number=w1450) -> (32bit integer=w1455:i32)
          n241 = Index Array(array=w1452, index=w1469) -> (element=w1472:dbl)
          n242 = Index Array(array=w1452, index=w1453) -> (element=w1454:dbl)
          n243 = case shown="0, Default" w1473 {
            tunnel: w1472 -> [w1507 w1509 w1513 w1516 w1519 w1522]
            tunnel: w1470 -> [w1506 w1510 w1512 w1515 w1518 w1521]
            tunnel: [w1505 w1508 w1511 w1514 w1517 w1520] -> w1447
            frame 0, Default {
              n244 = Less?(x=w1507, y=w1506) -> (x < y?=w1505:bool)
            }
            frame 1 {
              n245 = Less Or Equal?(x=w1509, y=w1510) -> (x <= y?=w1508:bool)
            }
            frame 2 {
              n246 = Equal?(x=w1513, y=w1512) -> (x = y?=w1511:bool)
            }
            frame 3 {
              n247 = Greater Or Equal?(x=w1516, y=w1515) -> (x >= y?=w1514:bool)
            }
            frame 4 {
              n248 = Greater?(x=w1519, y=w1518) -> (0:w1517:bool)
            }
            frame 5 {
              n249 = Not Equal?(x=w1522, y=w1521) -> (x != y?=w1520:bool)
            }
          }
          n250 = case shown="0, Default" w1455 {
            tunnel: w1454 -> [w1480 w1482 w1486 w1489 w1492 w1495]
            tunnel: w1449 -> [w1479 w1483 w1485 w1488 w1491 w1494]
            tunnel: [w1478 w1481 w1484 w1487 w1490 w1493] -> w1448
            frame 0, Default {
              n251 = Less?(x=w1480, y=w1479) -> (x < y?=w1478:bool)
            }
            frame 1 {
              n252 = Less Or Equal?(x=w1482, y=w1483) -> (x <= y?=w1481:bool)
            }
            frame 2 {
              n253 = Equal?(x=w1486, y=w1485) -> (x = y?=w1484:bool)
            }
            frame 3 {
              n254 = Greater Or Equal?(x=w1489, y=w1488) -> (x >= y?=w1487:bool)
            }
            frame 4 {
              n255 = Greater?(x=w1492, y=w1491) -> (0:w1490:bool)
            }
            frame 5 {
              n256 = Not Equal?(x=w1495, y=w1494) -> (x != y?=w1493:bool)
            }
          }
          n257 = And(x=w1447, y=w1448) -> (x .and. y?=w1446:bool)
          n258 = case shown="True" w1446 {
            tunnel: w1465 -> [w1497 w1504]
            tunnel: w1464 -> [w1496 w1503]
            tunnel: w1463 -> [_ w1502]
            tunnel: w1446 -> [_ w1501]
            tunnel: w1462 -> [_ w1500]
            tunnel: [w1496 w1499] -> w1461
            tunnel: [w1497 w1498] -> w1460
            frame False {
            }
            frame True {
              n259 = Replace Array Subset(array=w1504, new element=w1501, index=w1502) -> (w1498:bool[])
              n260 = Replace Array Subset(array=w1503, new element=w1500, index=w1502) -> (w1499:dbl[])
            }
          }
        }
        n261 = global write "gvbooleschRT.vi" "global stop RT"("global stop RT") -> ()
        n262 = Split 1D Array ("DIO")(array=w1406, index=w1391) -> (first subarray=w1405:dbl[], second subarray=w1403:dbl[])
        n263 = Split 1D Array "DIO"(array=w1412, index=w1391) -> (first subarray=w1378:bool[], second subarray=w1411:bool[])
        n264 = Split 1D Array(array=w1403, index=w1404) -> (first subarray=w1401:dbl[], second subarray=w1387:dbl[])
        n265 = Split 1D Array "FPGABoolesch"(array=w1411, index=w1404) -> (first subarray=→"ZwangsFPGABoolesch?":bool[], second subarray=w1389:bool[])
        n266 = Split 1D Array "Methodenübergreifend"(array=w1389, index=w1385) -> (first subarray=w1382:bool[], second subarray=w1388:bool[])
        n267 = Split 1D Array "LangsameHeizungen"(array=w1388, index=w1399) -> (first subarray=→"ZwangsLangsameH?":bool[], second subarray=w1410:bool[])
        n268 = Split 1D Array "BronkhorstSP"(array=w1410, index=w1397) -> (first subarray=w1408:bool[])  [unwired: 1 out]
        n269 = Split 1D Array(array=w1387, index=w1385) -> (first subarray=w1379:dbl[], second subarray=w1386:dbl[])
        n270 = Split 1D Array(array=w1386, index=w1399) -> (first subarray=w1394:dbl[], second subarray=w1398:dbl[])
        n271 = Split 1D Array(array=w1398, index=w1397) -> (first subarray=w1396:dbl[])  [unwired: 1 out]
        n272 = for {
          tunnel: [w1438] -> w1377 mode=indexing
          tunnel: w1392 -> [w1440] mode=indexing
          tunnel: [w1436] -> w1376 mode=indexing
          shift-right: [w1444] -> _
          shift-left: w1378 -> [w1445]
          shift-right: [w1442] -> _
          shift-left: w1405 -> [w1443]
          n273 = Split 1D Array(array=w1443, index=w1440) -> (first subarray=w1441:dbl[], second subarray=w1442:dbl[])
          n274 = Split 1D Array(array=w1445, index=w1440) -> (first subarray=w1439:bool[], second subarray=w1444:bool[])
          n275 = Greater Than 0?(x=w1441) -> (x > 0?=w1437:bool[])
          n276 = Bundle(w1439) -> (w1438:cluster{bool[]})  [unwired: 1 in]
          n277 = Bundle(w1437) -> (w1436:cluster{bool[]})  [unwired: 1 in]
        }
        "ZwangsDIO?" <- w1377
        "ZwangsDIO!" <- w1376
        n278 = for {
          tunnel: w1409 -> [w1432] mode=indexing
          shift-right: [w1434] -> _
          shift-left: w1408 -> [w1435]
          tunnel: [w1429] -> w1375 mode=indexing
          shift-right: [w1431] -> _
          shift-left: w1396 -> [w1433]
          tunnel: [w1427] -> w1374 mode=indexing
          n279 = Split 1D Array(array=w1435, index=w1432) -> (first subarray=w1430:bool[], second subarray=w1434:bool[])
          n280 = Split 1D Array(array=w1433, index=w1432) -> (first subarray=w1428:dbl[], second subarray=w1431:dbl[])
          n281 = Bundle(w1430) -> (w1429:cluster{bool[]})  [unwired: 1 in]
          n282 = Bundle(w1428) -> (w1427:cluster{dbl[]})  [unwired: 1 in]
        }
        "ZwangsHorst?" <- w1375
        "ZwangsHorst!" <- w1374
        n283 = Greater Than 0?(x=w1401) -> (x > 0?=→"ZwangsFPGABoolesch!":bool[])
        n284 = Index Array(array=w1382, index=0 ("Index")) -> (element=w1383:bool)
        n285 = Greater Than 0?(x=w1394) -> (x > 0?=→"ZwangsLangsameH!":bool[])
        n286 = Index Array(array=w1382, index=1 ("Index")) -> (element=w1380:bool)
        n287 = case shown="True" w1383 {
          tunnel: w1379 -> [_ w1425]
          frame False {
          }
          frame True {
            n288 = Index Array(array=w1425, index=0 ("Index")) -> (element=w1424:dbl)
            n289 = To Long Integer(number=w1424) -> (32bit integer=w1423:i32)
            n290 = local write "Methodennummer"(w1423) -> ()
          }
        }
        n291 = case shown="True" w1380 {
          tunnel: w1379 -> [_ w1422]
          frame False {
          }
          frame True {
            n292 = Index Array(array=w1422, index=1 ("Index")) -> (element=w1420:dbl)
            n293 = Greater Than 0?(x=w1420) -> (x > 0?=w1419:bool)
            n294 = local write "global stop RT"(w1419) -> ()
          }
        }
      }
      n295 = for {
        N: 1 -> [_]
        tunnel: w350 -> [w422]
        tunnel: [w422] -> w349
        n296 = call "Warten8"("Count(mSec)"=u32 100) -> ()  [unwired: 1 out]
      }
      n297 = while {
        shift-right: [w445] -> _
        shift-left: w352 -> [w444]
        tunnel: w355 -> [w443]
        tunnel: w357 -> [w442]
        tunnel: w358 -> [w428]
        shift-right: [w429] -> _
        shift-left: _ -> [w441]
        shift-right: [w439] -> _
        shift-left: w352 -> [w440]
        shift-right: [w436] -> _
        shift-left: 0 ("Index") -> [w438]
        tunnel: w349 -> [w437]
        tunnel: w356 -> [w435]
        shift-right: [w427] -> _
        shift-left: w353 -> [w434]
        tunnel: w354 -> [_]
        tunnel: i16[] [4, 4, 4, 4, 2, 4] -> [w425]
        i -> [w433]
        stop <- w424 stop-if-true
        n298 = local read "HorstSP"() -> (w445:dbl[])
        n299 = Not Equal?(x=w445, y=w444) -> (x != y?=w446:bool)
        n300 = case shown="False" w446 {
          tunnel: w445 -> [_ w529]
          tunnel: w444 -> [_ w528]
          tunnel: w443 -> [_ w527]
          tunnel: w442 -> [_ w526]
          tunnel: w428 -> [w473 w525]
          tunnel: [w472 w524] -> w429
          tunnel: w441 -> [w474 w523]
          tunnel: w440 -> [w469 w522]
          tunnel: [w469 w521] -> w439
          tunnel: w438 -> [w468 w520]
          tunnel: w437 -> [w482 _]
          tunnel: [w481 w520] -> w436
          tunnel: w435 -> [w475 _]
          tunnel: w434 -> [w471 w519]
          tunnel: [w470 w519] -> w427
          tunnel: w425 -> [_ w518]
          frame False {
            n301 = local read "Big Ben"() -> (w478:dbl)
            n302 = Index Array(array=w469, index=w468) -> (element=w480:dbl)
            n303 = Add(x=w480, y="Wartezeit nach SP(s)") -> (x+y=w477:dbl)
            n304 = Greater Or Equal?(x=w478, y=w477) -> (x >= y?=w476:bool)
            n305 = case shown="True" w476 {
              tunnel: w475 -> [_ w501]
              tunnel: w468 -> [_ w489]
              tunnel: w474 -> [w485 w497]
              tunnel: w473 -> [_ w496]
              tunnel: [w485 w491] -> w472
              tunnel: w471 -> [w486 w490]
              tunnel: [w486 w487] -> w470
              frame False {
              }
              frame True {
                n306 = Index Array(array=w501, index=w489) -> (element=w499:string)
                n307 = Replace Array Subset(array=w490, new element=w488, index=w489) -> (w487:string[])
                n308 = Concatenate Strings(w499, "\r\n") -> (w498:string)
                n309 = flat-sequence {
                  tunnel: w498 -> [w509]
                  tunnel: w497 -> [w508]
                  tunnel: w496 -> [w506]
                  tunnel: [w504] -> w494
                  tunnel: [w503] -> w492
                  tunnel: [w512] -> w495
                  tunnel: w494 -> [w512]
                  tunnel: [w511] -> w493
                  tunnel: w492 -> [w511]
                  tunnel: w495 -> [w515]
                  tunnel: w493 -> [w516]
                  tunnel: [w514] -> w491
                  tunnel: [w513] -> w488
                  frame #0 {
                    n310 = call "serialwritefpga.vi"("FPGA VI Reference In"=w506, "Port"=T9."1", "String"=w509, "error in"=w508, 4:TRUE ("write"), 7:1 ("Timeout (ms)")) -> ("FPGA VI Reference Out"=w503:refnum<k20>, "error out"=w504:errorcluster)
                  }
                  frame #1 {
                    n311 = call "Warten23"("Count(mSec)"="Wartezeit nach MW(ms)") -> ()  [unwired: 1 out]
                  }
                  frame #2 {
                    n312 = call "serialreadfpga.vi"("error in"=w515, "Timeout (ms)"=1, "FPGA VI Reference In"=w516) -> ("Port1"=w513:string, "error out"=w514:errorcluster)  [unwired: 3 in, 8 out]
                  }
                }
              }
            }
            n313 = Add(x=w468, y=1) -> (x+y=w483:i32)
            n314 = Quotient & Remainder(x=w483, y=w482) -> (x-y*floor(x/y)=w481:i32)  [unwired: 1 out]
          }
          frame True {
            n315 = for {
              tunnel: w529 -> [w539] mode=indexing
              tunnel: w528 -> [w540] mode=indexing
              tunnel: w527 -> [w538] mode=indexing
              tunnel: w526 -> [w537] mode=indexing
              tunnel: w525 -> [w536]
              tunnel: [w534] -> w524
              tunnel: w523 -> [w533]
              tunnel: w522 -> [w532] mode=indexing
              tunnel: [w531] -> w521 mode=indexing
              tunnel: w518 -> [w530] mode=indexing
              n316 = Not Equal?(x=w539, y=w540) -> (x != y?=w535:bool)
              n317 = case shown="True" w535 {
                tunnel: w539 -> [_ w556]
                tunnel: w538 -> [_ w557]
                tunnel: w537 -> [_ w553]
                tunnel: w536 -> [_ w550]
                tunnel: [w542 w547] -> w534
                tunnel: w533 -> [w542 w546]
                tunnel: w532 -> [w541 _]
                tunnel: [w541 w545] -> w531
                tunnel: w530 -> [_ w543]
                frame False {
                }
                frame True {
                  n318 = Divide(x=w556, y=w557) -> (x/y=w555:dbl)
                  n319 = To Long Integer(number=w555) -> (32bit integer=w554:i32)
                  n320 = local read "Big Ben"() -> (w545:dbl)
                  n321 = Number To Hexadecimal String(1:w543, 2:w554) -> (0:w559:string)
                  n322 = call "Warten7"("Count(mSec)"="nach sp warten(ms)") -> ()  [unwired: 1 out]
                  n323 = Concatenate Strings(w553, w559, "\r\n") -> (w552:string)
                  n324 = call "serialwritefpga.vi"("FPGA VI Reference In"=w550, "Port"=T9."1", "String"=w552, "error in"=w546, 4:TRUE ("write"), 7:1 ("Timeout (ms)")) -> ("error out"=w547:errorcluster)  [unwired: 1 out]
                }
              }
            }
          }
        }
        "RS232 Array" <- w427
        n325 = global read "gvbooleschRT.vi" "global stop RT"() -> (w424:bool)
        n326 = xnode "Read/Write Control"("FPGA VI Reference In"=w428, "error in"=w429) -> ("error out"=w432:errorcluster, "Error Out"=w431)  [unwired: 1 out]
        n327 = Concatenate Strings(w427) -> (→"RS-232":string)
        n328 = Merge Errors(w432, w431) -> (w430:errorcluster)
        n329 = Unbundle By Name(w430) -> ("status"=→"status":bool)
        "Zähler serielle Kommunikation" <- w433
        "Array" <- w440
      }
      n330 = while "AIMittelwerte" {
        tunnel: w358 -> [w1107]
        tunnel: w411 -> [w1098]
        tunnel: w409 -> [w1097]
        tunnel: w407 -> [w1093]
        tunnel: w403 -> [w1086]
        tunnel: w402 -> [w1084]
        tunnel: w401 -> [w1083]
        tunnel: w397 -> [w1076]
        tunnel: w396 -> [w1075]
        tunnel: w395 -> [w1074]
        tunnel: w383 -> [w1057]
        tunnel: w382 -> [w1056]
        tunnel: w381 -> [w1055]
        stop <- w1112 stop-if-true
        w1063 = 10.0
        n331 = xnode "Read/Write Control"("FPGA VI Reference In"=w1107) -> ("Mod1/AI"=w1106:void[], "Mod2/AI"=w1105:void[], "Mod3/AI"=w1104:void[], "UWidr[V]Trap1"=w1072, "UTemp[V]Trap1"=w1071, "UWidr[V]Trap2"=w1070, "UTemp[V]Trap2"=w1069, "U[V]Mach1"=w1068, "U[V]Mach2"=w1067)  [unwired: 1 in, 2 out]
        n332 = call "Warten26"("Count(mSec)"=u32 100) -> ()  [unwired: 1 out]
        n333 = To Double Precision Float(number=w1106) -> (double precision float=w1103:dbl[])
        n334 = To Double Precision Float(number=w1105) -> (double precision float=w1102:dbl[])
        n335 = To Double Precision Float(number=w1104) -> (double precision float=w1101:dbl[])
        n336 = Build Array(w1072, w1071, w1070, w1069, w1068, w1067) -> (w1066:void[])
        n337 = To Double Precision Float(number=w1066) -> (double precision float=w1065:dbl[])
        n338 = for {
          N: 9 -> [_]
          shift-right: [w1179] -> w1110
          shift-left: w1103 -> [w1182]
          shift-right: [w1178] -> w1109
          shift-left: w1102 -> [w1181]
          shift-right: [w1177] -> w1108
          shift-left: w1101 -> [w1180]
          tunnel: w1107 -> [w1176]
          shift-right: [w1174] -> w1064
          shift-left: w1065 -> [w1175]
          n339 = flat-sequence {
            tunnel: w1182 -> [w1200]
            tunnel: w1181 -> [w1199]
            tunnel: w1180 -> [w1198]
            tunnel: [w1197] -> w1179
            tunnel: [w1196] -> w1178
            tunnel: [w1195] -> w1177
            tunnel: w1176 -> [w1194]
            tunnel: w1175 -> [w1185]
            tunnel: [w1184] -> w1174
            frame #0 {
              n340 = call "Warten4"("Count(mSec)"=u32 10) -> ()  [unwired: 1 out]
            }
            frame #1 {
              n341 = xnode "Read/Write Control"("FPGA VI Reference In"=w1194) -> ("Mod1/AI"=w1204:void[], "Mod2/AI"=w1205:void[], "Mod3/AI"=w1206:void[], "UWidr[V]Trap1"=w1193, "UTemp[V]Trap1"=w1192, "UWidr[V]Trap2"=w1191, "UTemp[V]Trap2"=w1190, "U[V]Mach1"=w1189, "U[V]Mach2"=w1188)  [unwired: 1 in, 2 out]
              n342 = Build Array(w1193, w1192, w1191, w1190, w1189, w1188) -> (w1187:void[])
              n343 = To Double Precision Float(number=w1204) -> (double precision float=w1203:dbl[])
              n344 = To Double Precision Float(number=w1205) -> (double precision float=w1202:dbl[])
              n345 = To Double Precision Float(number=w1206) -> (double precision float=w1201:dbl[])
              n346 = To Double Precision Float(number=w1187) -> (double precision float=w1186:dbl[])
              n347 = Add(x=w1200, y=w1203) -> (x+y=w1197:dbl[])
              n348 = Add(x=w1199, y=w1202) -> (x+y=w1196:dbl[])
              n349 = Add(x=w1198, y=w1201) -> (x+y=w1195:dbl[])
              n350 = Add(x=w1185, y=w1186) -> (x+y=w1184:dbl[])
            }
          }
        }
        n351 = Divide(x=w1064, y=w1063) -> (x/y=w1062:dbl[])
        n352 = Divide(x=w1110, y=w1063) -> (x/y=w1096:dbl[])
        n353 = Divide(x=w1109, y=w1063) -> (x/y=w1085:dbl[])
        n354 = Divide(x=w1108, y=w1063) -> (x/y=w1079:dbl[])
        n355 = Square(x=w1062) -> (x^2=w1061:dbl[])
        n356 = Multiply(x=w1061, y=w1057) -> (x*y=w1060:dbl[])
        n357 = Multiply(x=w1062, y=w1056) -> (x*y=w1059:dbl[])
        n358 = Multiply(x=w1096, y=w1097) -> (x*y=w1094:dbl[])
        n359 = Multiply(x=w1085, y=w1084) -> (x*y=w1088:dbl[])
        n360 = Multiply(x=w1079, y=w1075) -> (x*y=w1077:dbl[])
        n361 = Square(x=w1096) -> (x^2=w1099:dbl[])
        n362 = Square(x=w1085) -> (x^2=w1090:dbl[])
        n363 = Square(x=w1079) -> (x^2=w1080:dbl[])
        n364 = Add(x=w1060, y=w1059) -> (x+y=w1058:dbl[])
        n365 = Multiply(x=w1099, y=w1098) -> (x*y=w1095:dbl[])
        n366 = Multiply(x=w1090, y=w1086) -> (x*y=w1089:dbl[])
        n367 = Multiply(x=w1080, y=w1076) -> (x*y=w1078:dbl[])
        n368 = Add(x=w1058, y=w1055) -> (x+y=→"Traps/Machs":dbl[])
        n369 = Add(x=w1095, y=w1094) -> (x+y=w1092:dbl[])
        n370 = Add(x=w1089, y=w1088) -> (x+y=w1087:dbl[])
        n371 = Add(x=w1078, y=w1077) -> (x+y=w1081:dbl[])
        n372 = Add(x=w1092, y=w1093) -> (x+y=→"Mod1/AI":dbl[])
        n373 = Add(x=w1087, y=w1083) -> (x+y=→"Mod2/AI":dbl[])
        n374 = Add(x=w1081, y=w1074) -> (x+y=→"Mod3/AI":dbl[])
        n375 = global read "gvbooleschRT.vi" "global stop RT"() -> (w1112:bool)
      }
      n376 = while "Methoden- und Zyklussteuerung" {
        shift-right: [w1589] -> _
        shift-left: 0.0 -> [w1588]
        shift-right: [w1587] -> _
        shift-left: -1 -> [w1586]
        tunnel: w358 -> [w1576]
        tunnel: w380 -> [w1580]
        tunnel: w389 -> [w1579]
        tunnel: w375 -> [w1569]
        tunnel: w363 -> [w1568]
        i -> [w1592]
        stop <- w1593 stop-if-true
        w1570 = 0  # ZeileMach2
        w1571 = 0  # ZeileMach1
        w1572 = 0  # ZeileFPGAFixp
        w1573 = 0  # ZeileFPGAPID
        w1575 = 0  # ZeileFPGABoolesch
        w1578 = i32[] [0, 0, 0, 0]  # ZeilennummernHorst
        w1583 = i32[] [0, 0, 0, 0]  # ZeilennummernDIOs
        n377 = local read "veränderte Methode benutzen"() -> (w1523:bool)
        n378 = local read "Methodennummer"() -> (w1567:i32)
        n379 = Index Array(array=w1568, index=w1567) -> (element=w1525:T2)
        n380 = case shown="True" w1523 {
          tunnel: w1525 -> [w1594 _]
          tunnel: [w1594 w1596] -> w1524
          frame False {
          }
          frame True {
            n381 = local read "veränderte Methode"() -> (w1596:T2)
            n382 = property on="veränderte Methode benutzen" class="Bool (strict)"("Value"=FALSE ("Methode verändern")) -> ()  [unwired: 2 in, 2 out]
          }
        }
        n383 = Unbundle(w1524) -> ("Zykluslängen [s]"=w1566:dbl[], "ZeitpktDIOsMod0"=w1536:dbl[], "ZeitpktDIOsMod1"=w1535:dbl[], "ZeitpktDIOsMod2A"=w1534:dbl[], "ZeitpktDIOsMod2B"=w1533:dbl[], "DIOsSPMod0"=w1541:bool[][], "DIOsSPMod1"=w1540:bool[][], "DIOsSPMod2A"=w1539:bool[][], "DIOsSPMod2B"=w1538:bool[][], "Mod0HorstZeitpkt"=w1546:dbl[], "Mod1HorstZeitpkt"=w1545:dbl[], "Mod2AHorstZeitpkt"=w1544:dbl[], "Mod2BHorstZeitpkt"=w1543:dbl[], "HorstSPMod0"=w1551:dbl[][], "HorstSPMod1"=w1550:dbl[][], "HorstSPMod2A"=w1549:dbl[][], "HorstSPMod2B"=w1548:dbl[][], "LangsameHeizungenSP"=w1565:dbl[], "LHHeizen?"=w1564:bool[], "ZPktFPGABoolesch"=w1562:dbl[], "FPGABoolesch"=w1561:bool[][], "ZeitpktFPGAPID"=w1560:dbl[], "FPGAPID"=w1559:T25, "ZeitpktFPGAFixp"=w1558:dbl[], "FPGAFixp"=w1557:fxp<+/-,16,4>[][], "ZeitpktMach1"=w1556:dbl[], "TempMach1"=w1555:dbl[], "ZeitpktMach2"=w1554:dbl[], "TempMach2"=w1553:dbl[], "PIDs für \"träge\" Heizungen"=→"PIDs für \"träge\" Heizungen":T3, "Zwangsbedingungen"=→"Zwangsbedingungen":dbl[][], "Text0 MS-Datei"=w1531:string, "Info"=w1530:string, "wie wird gespeichert?"=w1529:u16, "Speicherlänge"=w1528:string, "Dateien fürs MS schicken?"=w1527:bool, "Pfad MS-Datei CRIO"=w1526:path)
        "Zykluslängen [s]" <- w1566
        n384 = local write "LangsameHeizungenSP"(w1565) -> ()
        n385 = local write "Text0 MS-Datei"(w1531) -> ()
        n386 = local write "wie wird gespeichert?"(w1529) -> ()
        n387 = Build Cluster Array(w1546, w1545, w1544, w1543) -> (w1542:cluster{"Mod2BHorstZeitpkt":dbl[]}[])
        n388 = Build Cluster Array(w1551, w1550, w1549, w1548) -> (w1547:cluster{"HorstSPMod2B":dbl[][]}[])
        n389 = Build Cluster Array(w1541, w1540, w1539, w1538) -> (w1537:cluster{"DIOsSPMod2B":bool[][]}[])
        n390 = local write "Speicherlänge"(w1528) -> ()
        n391 = local write "Info"(w1530) -> ()
        n392 = local write "Pfad MS-Datei CRIO"(w1526) -> ()
        n393 = local write "Dateien fürs MS schicken?"(w1527) -> ()
        n394 = Build Cluster Array(w1536, w1535, w1534, w1533) -> (w1532:cluster{"ZeitpktDIOsMod2B":dbl[]}[])
        n395 = Add(x=w1586, y=1) -> (x+y=w1584:i32)
        n396 = local read "Zyklusnummern 0, 1, 2A, 2B"() -> (w1582:i32[])
        n397 = local read "ZwangsFPGABoolesch?"() -> (w1574:bool[])
        n398 = local read "ZwangsHorst?"() -> (w1577:cluster{bool[]}[])
        n399 = local read "ZwangsDIO?"() -> (w1581:cluster{bool[]}[])
        n400 = while "ZyklusSteuerung" {
          shift-right: [w1753] -> _
          shift-left: w1582 -> [w1752]
          shift-right: [w1745] -> _
          shift-left: w1583 -> [w1750]
          tunnel: w1532 -> [w1748]
          shift-right: [w1604] -> _
          shift-left: w1581 -> [w1605]
          tunnel: w1537 -> [w1602]
          tunnel: w1580 -> [w1739]
          tunnel: w1579 -> [w1738]
          tunnel: w1576 -> [w1660]
          tunnel: w1542 -> [w1736]
          shift-right: [w1733] -> _
          shift-left: w1578 -> [w1737]
          shift-right: [w1607] -> _
          shift-left: w1577 -> [w1608]
          tunnel: w1547 -> [w1611]
          shift-right: [w1720] -> _
          shift-left: w1575 -> [w1726]
          tunnel: w1562 -> [w1727]
          tunnel: w1561 -> [w1713]
          shift-right: [w1714] -> _
          shift-left: w1574 -> [w1718]
          tunnel: w1560 -> [w1711]
          shift-right: [w1707] -> _
          shift-left: w1573 -> [w1712]
          tunnel: w1559 -> [w1705]
          shift-right: [w1698] -> _
          shift-left: w1572 -> [w1703]
          tunnel: w1558 -> [w1702]
          tunnel: w1557 -> [w1696]
          shift-right: [w1683] -> _
          shift-left: w1571 -> [w1694]
          tunnel: w1556 -> [w1692]
          tunnel: w1555 -> [w1691]
          shift-right: [w1627] -> _
          shift-left: w1570 -> [w1629]
          tunnel: w1554 -> [w1626]
          tunnel: w1553 -> [w1625]
          tunnel: w1569 -> [_]
          tunnel: w1564 -> [w1622]
          stop <- w1598 stop-if-true
          w1632 = 6.0782 ("y")
          w1665 = 6.0782 ("y")
          n401 = local read "ZwangsHorst?"() -> (w1607:cluster{bool[]}[])
          n402 = local read "ZwangsFPGABoolesch?"() -> (w1714:bool[])
          n403 = local read "Zyklusnummern 0, 1, 2A, 2B"() -> (w1753:i32[])
          n404 = local read "ZwangsDIO?"() -> (w1604:cluster{bool[]}[])
          n405 = Not Equal?(x=w1714, y=w1718) -> (x != y?=w1717:bool)
          n406 = Not Equal?(x=w1605, y=w1604) -> (x != y?=w1603:bool)
          n407 = Equal?(x=w1753, y=w1752) -> (x = y?=w1751:bool[])
          n408 = local read "ZwangsLangsameH?"() -> (w1620:bool[])
          n409 = Not Equal?(x=w1607, y=w1608) -> (x != y?=w1606:bool)
          n410 = local read "ZwangsLangsameH!"() -> (w1619:bool[])
          n411 = Boolean To (0,1)(Boolean=w1751) -> (0, 1=w1749:i16[])
          n412 = To Long Integer(number=w1749) -> (32bit integer=w1729:i32[])
          n413 = Multiply(x=w1729, y=w1737) -> (x*y=w1609:i32[])
          n414 = Index Array(array=w1729, index=1 ("Index")) -> (element=w1628:i32)
          n415 = Multiply(x=w1628, y=w1694) -> (x*y=w1684:i32)
          n416 = Multiply(x=w1628, y=w1703) -> (x*y=w1697:i32)
          n417 = Multiply(x=w1628, y=w1629) -> (x*y=w1652:i32)
          n418 = Add(x=1 ("y"), y=w1684) -> (x+y=w1690:i32)
          n419 = Index Array(array=w1702, index=w1697) -> (element=w1701:dbl)
          n420 = Add(x=1 ("y"), y=w1652) -> (x+y=w1658:i32)
          n421 = Multiply(x=w1628, y=w1712) -> (x*y=w1704:i32)
          n422 = Index Array(array=w1692, index=w1684) -> (element=w1682:dbl)
          n423 = Index Array(array=w1692, index=w1690) -> (element=w1688:dbl)
          n424 = Multiply(x=w1628, y=w1726) -> (x*y=w1715:i32)
          n425 = Index Array(array=w1727, index=w1715) -> (element=w1723:dbl)
          n426 = Index Array(array=w1691, index=w1684) -> (element=w1676:dbl)
          n427 = Index Array(array=w1691, index=w1690) -> (element=w1689:dbl)
          n428 = Index Array(array=w1626, index=w1652) -> (element=w1651:dbl)
          n429 = Index Array(array=w1626, index=w1658) -> (element=w1656:dbl)
          n430 = Index Array(array=w1625, index=w1652) -> (element=w1645:dbl)
          n431 = Index Array(array=w1625, index=w1658) -> (element=w1657:dbl)
          n432 = Index Array(array=w1711, index=w1704) -> (element=w1710:dbl)
          n433 = Subtract(x=w1688, y=w1682) -> (x-y=w1680:dbl)
          n434 = Subtract(x=w1689, y=w1676) -> (x-y=w1678:dbl)
          n435 = Subtract(x=w1656, y=w1651) -> (x-y=w1649:dbl)
          n436 = Subtract(x=w1657, y=w1645) -> (x-y=w1647:dbl)
          n437 = Multiply(x=w1729, y=w1750) -> (x*y=w1613:i32[])
          n438 = Not(x=w1620) -> (.not. x?=w1621:bool[])
          n439 = local read "Zykluszeiten 0, 1, 2A, 2B"() -> (w1725:dbl[])
          n440 = Index Array(array=w1725, index=1 ("Index")) -> (element=w1624:dbl)
          n441 = Greater Or Equal?(x=w1624, y=w1701) -> (x >= y?=w1695:bool)
          n442 = Boolean To (0,1)(Boolean=w1695) -> (0, 1=w1700:i16)
          n443 = Greater Or Equal?(x=w1624, y=w1688) -> (x >= y?=w1687:bool)
          n444 = To Long Integer(number=w1700) -> (32bit integer=w1699:i32)
          n445 = Greater Or Equal?(x=w1624, y=w1656) -> (x >= y?=w1655:bool)
          n446 = Greater Or Equal?(x=w1624, y=w1710) -> (x >= y?=w1706:bool)
          n447 = Subtract(x=w1624, y=w1682) -> (x-y=w1681:dbl)
          n448 = Greater Or Equal?(x=w1624, y=w1723) -> (x >= y?=w1719:bool)
          n449 = Boolean To (0,1)(Boolean=w1687) -> (0, 1=w1686:i16)
          n450 = Subtract(x=w1624, y=w1651) -> (x-y=w1650:dbl)
          n451 = Add(x=w1697, y=w1699) -> (x+y=w1698:i32)
          n452 = Boolean To (0,1)(Boolean=w1655) -> (0, 1=w1654:i16)
          n453 = Boolean To (0,1)(Boolean=w1706) -> (0, 1=w1709:i16)
          n454 = Divide(x=w1681, y=w1680) -> (x/y=w1679:dbl)
          n455 = Boolean To (0,1)(Boolean=w1719) -> (0, 1=w1722:i16)
          n456 = To Long Integer(number=w1686) -> (32bit integer=w1685:i32)
          n457 = Or(x=w1719, y=w1717) -> (x .or. y?=w1716:bool)
          n458 = for {
            tunnel: w1609 -> [w1994] mode=indexing
            tunnel: w1725 -> [w1993] mode=indexing
            tunnel: w1736 -> [w1990] mode=indexing
            tunnel: [w1991] -> w1610 mode=indexing
            n459 = Unbundle(w1990) -> ("Mod2BHorstZeitpkt"=w1989:dbl[])
            n460 = Index Array(array=w1989, index=w1994) -> (element=w1992:dbl)
            n461 = Greater Or Equal?(x=w1993, y=w1992) -> (x >= y?=w1991:bool)
          }
          n462 = Divide(x=w1650, y=w1649) -> (x/y=w1648:dbl)
          n463 = Multiply(x=w1679, y=w1678) -> (x*y=w1677:dbl)
          n464 = To Long Integer(number=w1709) -> (32bit integer=w1708:i32)
          n465 = To Long Integer(number=w1654) -> (32bit integer=w1653:i32)
          n466 = And(x=w1620, y=w1619) -> (x .and. y?=w1617:bool[])
          n467 = for {
            tunnel: w1613 -> [w2067] mode=indexing
            tunnel: w1725 -> [w2066] mode=indexing
            tunnel: [w2065] -> w1601 mode=indexing
            tunnel: w1748 -> [w2063] mode=indexing
            n468 = Unbundle(w2063) -> ("ZeitpktDIOsMod2B"=w2062:dbl[])
            n469 = Index Array(array=w2062, index=w2067) -> (element=w2064:dbl)
            n470 = Greater Or Equal?(x=w2066, y=w2064) -> (x >= y?=w2065:bool)
          }
          n471 = To Long Integer(number=w1722) -> (32bit integer=w1721:i32)
          n472 = Add(x=w1677, y=w1676) -> (x+y=w1662:dbl)
          n473 = Multiply(x=w1648, y=w1647) -> (x*y=w1646:dbl)
          n474 = And(x=w1621, y=w1622) -> (x .and. y?=w1618:bool[])
          n475 = Add(x=w1684, y=w1685) -> (x+y=w1683:i32)
          n476 = Add(x=w1704, y=w1708) -> (x+y=w1707:i32)
          n477 = case shown="True" w1695 {
            tunnel: w1697 -> [_ w1812]
            tunnel: w1696 -> [_ w1824]
            tunnel: w1660 -> [_ w1814]
            frame False {
            }
            frame True {
              n478 = Index Array(array=w1824, index (row)=w1812) -> (element=w1813:fxp<+/-,16,4>[])  [unwired: 1 in]
              n479 = Array To Cluster(array=w1813) -> (cluster=w1823:T26)
              n480 = Unbundle(w1823) -> ("FPGAFixp[0]"=w1822:fxp<+/-,16,4>, "FPGAFixp[1]"=w1821:fxp<+/-,16,4>, "FPGAFixp[2]"=w1820:fxp<+/-,16,4>, "FPGAFixp[3]"=w1819:fxp<+/-,16,4>, "FPGAFixp[4]"=w1818:fxp<+/-,16,4>, "FPGAFixp[5]"=w1817:fxp<+/-,16,4>, "FPGAFixp[6]"=w1816:fxp<+/-,16,4>, "FPGAFixp[7]"=w1815:fxp<+/-,16,4>)
              n481 = xnode "Read/Write Control"("FPGA VI Reference In"=w1814, "UTempSPTrap1"=w1822, "UTempMaxTrap1"=w1821, "UWidrMaxTrap1"=w1820, "UTempSPTrap2"=w1819, "UTempMaxTrap2"=w1818, "UWidrMaxTrap2"=w1817, "Umax[V]Mach1"=w1816, "Umax[V]Mach2"=w1815) -> ()  [unwired: 1 in, 2 out]
            }
          }
          n482 = Add(x=w1646, y=w1645) -> (x+y=w1630:dbl)
          n483 = Add(x=w1652, y=w1653) -> (x+y=w1627:i32)
          n484 = Add(x=w1715, y=w1721) -> (x+y=w1720:i32)
          n485 = Or(x=w1618, y=w1617) -> (x .or. y?=w1616:bool[])
          n486 = local write "Heizen?LH"(w1616) -> ()
          n487 = case shown="True" w1706 {
            tunnel: w1660 -> [_ w1889]
            tunnel: w1705 -> [_ w1888]
            tunnel: w1704 -> [_ w1881]
            frame False {
            }
            frame True {
              n488 = Index Array(array=w1888, index (row)=w1881) -> (element=w1887:T27)  [unwired: 1 in]
              n489 = Array To Cluster(array=w1887) -> (cluster=w1886:T28)
              n490 = Unbundle(w1886) -> ("FPGAPID[0]"=w1885:T29, "FPGAPID[1]"=w1884:T29, "FPGAPID[2]"=w1883:T29, "FPGAPID[3]"=w1882:T29)
              n491 = xnode "Read/Write Control"("FPGA VI Reference In"=w1889, "PIDTrap1"=w1885, "PIDTrap2"=w1884, "PIDMach1"=w1883, "PIDMach2"=w1882) -> ()  [unwired: 1 in, 2 out]
            }
          }
          n492 = case shown="True" w1716 {
            tunnel: w1715 -> [_ w1926]
            tunnel: w1714 -> [_ w1937]
            tunnel: w1713 -> [_ w1942]
            tunnel: w1660 -> [_ w1934]
            frame False {
            }
            frame True {
              n493 = local read "ZwangsFPGABoolesch!"() -> (w1938:bool[])
              n494 = Index Array(array=w1942, index (row)=w1926) -> (element=w1940:bool[])  [unwired: 1 in]
              n495 = Not(x=w1937) -> (.not. x?=w1941:bool[])
              n496 = And(x=w1940, y=w1941) -> (x .and. y?=w1939:bool[])
              n497 = And(x=w1937, y=w1938) -> (x .and. y?=w1936:bool[])
              n498 = Or(x=w1939, y=w1936) -> (x .or. y?=w1935:bool[])
              n499 = Array To Cluster(array=w1935) -> (cluster=w1933:T30)
              n500 = Unbundle(w1933) -> ("[0]"=w1932:bool, "[1]"=w1931:bool, "[2]"=w1930:bool, "[3]"=w1929:bool, "[4]"=w1928:bool, "[5]"=w1927:bool)
              n501 = xnode "Read/Write Control"("FPGA VI Reference In"=w1934, "ServoTrap1kalt"=w1932, "ServoTrap2kalt"=w1931, "Heizen?Trap1"=w1930, "Heizen?Trap2"=w1929, "Heizen?Mach1"=w1928, "Heizen?Mach2"=w1927) -> ()  [unwired: 1 in, 2 out]
            }
          }
          n502 = Boolean To (0,1)(Boolean=w1610) -> (0, 1=w1735:i16[])
          n503 = Boolean Array To Number(Boolean array=w1610) -> (number=w1732:u32)
          n504 = Multiply(x=2.0, y=w1665) -> (x*y=w1673:dbl)
          n505 = Multiply(x=153.1621 ("y"), y=-1.0) -> (x*y=w1674:dbl)
          n506 = call "Warten13"("Count(mSec)"=u32 100) -> ()  [unwired: 1 out]
          n507 = Multiply(x=2.0 ("y"), y=w1632) -> (x*y=w1640:dbl)
          n508 = Multiply(x=153.1621 ("y"), y=-1.0) -> (x*y=w1642:dbl)
          n509 = To Long Integer(number=w1735) -> (32bit integer=w1734:i32[])
          n510 = Subtract(x=-237.2852 ("y"), y=w1662) -> (x-y=w1670:dbl)
          n511 = Greater?(x=w1732, y=u32 0) -> (0:w1730:bool)
          n512 = Or(x=w1730, y=w1606) -> (x .or. y?=w1612:bool)
          n513 = Divide(x=w1674, y=w1673) -> (x/y=w1667:dbl)
          n514 = Boolean To (0,1)(Boolean=w1601) -> (0, 1=w1747:i16[])
          n515 = Boolean Array To Number(Boolean array=w1601) -> (number=w1744:u32)
          n516 = Greater?(x=w1744, y=u32 0) -> (0:w1741:bool)
          n517 = Or(x=w1741, y=w1603) -> (x .or. y?=w1742:bool)
          n518 = case shown="True" w1742 {
            tunnel: w1613 -> [_ w2000]
            tunnel: w1604 -> [_ w1997]
            tunnel: w1739 -> [_ w2007]
            tunnel: w1738 -> [_ w2006]
            tunnel: w1660 -> [_ w2005]
            tunnel: w1602 -> [_ w1998]
            tunnel: w1601 -> [_ w1999]
            frame False {
            }
            frame True {
              n519 = local read "ZwangsDIO!"() -> (w1996:cluster{bool[]}[])
              n520 = for {
                tunnel: w2000 -> [w2022] mode=indexing
                tunnel: w1999 -> [w2021] mode=indexing
                tunnel: w1998 -> [w2020] mode=indexing
                tunnel: w1997 -> [w2019] mode=indexing
                tunnel: w1996 -> [w2018] mode=indexing
                tunnel: [w2008] -> w1995 mode=indexing
                n521 = Not(x=w2021) -> (.not. x?=w2024:bool)
                n522 = Unbundle(w2020) -> ("DIOsSPMod2B"=w2017:bool[][])
                n523 = Unbundle(w2019) -> (w2013:bool[])
                n524 = Unbundle(w2018) -> (w2012:bool[])
                n525 = Boolean To (0,1)(Boolean=w2024) -> (0, 1=w2023:i16)
                n526 = Not(x=w2013) -> (.not. x?=w2014:bool[])
                n527 = To Long Integer(number=w2023) -> (32bit integer=w2025:i32)
                n528 = Subtract(x=w2022, y=w2025) -> (x-y=w2016:i32)
                n529 = And(x=w2013, y=w2012) -> (x .and. y?=w2010:bool[])
                n530 = Index Array(array=w2017, index (row)=w2016) -> (element=w2015:bool[])  [unwired: 1 in]
                n531 = And(x=w2015, y=w2014) -> (x .and. y?=w2011:bool[])
                n532 = Or(x=w2011, y=w2010) -> (x .or. y?=w2009:bool[])
                n533 = Bundle(w2009) -> (w2008:cluster{bool[]})  [unwired: 1 in]
              }
              n534 = for {
                tunnel: w1995 -> [w2053] mode=indexing
                tunnel: w2007 -> [w2055] mode=indexing
                shift-right: [w2056] -> w2003
                shift-left: w2006 -> [w2057]
                n535 = Unbundle(w2053) -> (w2052:bool[])
                n536 = Unbundle(w2055) -> ("DIOsMod2BNr"=w2054:i32[])
                n537 = for {
                  tunnel: w2052 -> [w2059] mode=indexing
                  tunnel: w2054 -> [w2060] mode=indexing
                  shift-right: [w2058] -> w2056
                  shift-left: w2057 -> [w2061]
                  n538 = Replace Array Subset(array=w2061, new element=w2059, index=w2060) -> (w2058:bool[])
                }
              }
              n539 = Split 1D Array(array=w2003, index=32 ("Länge")) -> (first subarray=w2002:bool[], second subarray=w2001:bool[])
              n540 = xnode "Read/Write Control"("FPGA VI Reference In"=w2005, "Mod5/DIO"=w2002, "Mod6/DIO"=w2001) -> ()  [unwired: 1 in, 2 out]
            }
          }
          n541 = Subtract(x=-237.2852 ("y"), y=w1630) -> (x-y=w1637:dbl)
          n542 = Divide(x=w1642, y=w1640) -> (x/y=w1634:dbl)
          n543 = case shown="True" w1612 {
            tunnel: w1611 -> [_ w1759]
            tunnel: w1607 -> [_ w1760]
            tunnel: w1610 -> [_ w1762]
            tunnel: w1609 -> [_ w1761]
            frame False {
            }
            frame True {
              n544 = local read "ZwangsHorst!"() -> (w1758:cluster{dbl[]}[])
              n545 = for {
                tunnel: w1762 -> [w1782] mode=indexing
                tunnel: w1761 -> [w1779] mode=indexing
                tunnel: w1760 -> [w1785] mode=indexing
                tunnel: w1759 -> [w1783] mode=indexing
                tunnel: w1758 -> [w1784] mode=indexing
                shift-right: [w1763] -> w1756
                shift-left: dbl[] [] -> [w1765]
                n546 = Unbundle(w1783) -> ("HorstSPMod2B"=w1777:dbl[][])
                n547 = Unbundle(w1784) -> (w1768:dbl[])
                n548 = Unbundle(w1785) -> (w1772:bool[])
                n549 = Not(x=w1782) -> (.not. x?=w1781:bool)
                n550 = Not(x=w1772) -> (.not. x?=w1775:bool[])
                n551 = Boolean To (0,1)(Boolean=w1781) -> (0, 1=w1780:i16)
                n552 = To Long Integer(number=w1780) -> (32bit integer=w1778:i32)
                n553 = Boolean To (0,1)(Boolean=w1775) -> (0, 1=w1774:i16[])
                n554 = Boolean To (0,1)(Boolean=w1772) -> (0, 1=w1773:i16[])
                n555 = To Double Precision Float(number=w1774) -> (double precision float=w1770:dbl[])
                n556 = To Double Precision Float(number=w1773) -> (double precision float=w1769:dbl[])
                n557 = Subtract(x=w1779, y=w1778) -> (x-y=w1776:i32)
                n558 = Multiply(x=w1769, y=w1768) -> (x*y=w1766:dbl[])
                n559 = Index Array(array=w1777, index (row)=w1776) -> (element=w1771:dbl[])  [unwired: 1 in]
                n560 = Multiply(x=w1771, y=w1770) -> (x*y=w1767:dbl[])
                n561 = Add(x=w1767, y=w1766) -> (x+y=w1764:dbl[])
                n562 = Build Array (concatenate)(w1765, w1764) -> (w1763:dbl[])
              }
              "HorstSP" <- w1756
            }
          }
          n563 = Add(x=w1609, y=w1734) -> (x+y=w1733:i32[])
          n564 = Square(x=w1667) -> (x^2=w1672:dbl)
          n565 = Divide(x=w1670, y=w1665) -> (x/y=w1669:dbl)
          n566 = To Long Integer(number=w1747) -> (32bit integer=w1746:i32[])
          n567 = Square(x=w1634) -> (x^2=w1639:dbl)
          n568 = Divide(x=w1637, y=w1632) -> (x/y=w1636:dbl)
          n569 = Subtract(x=w1672, y=w1669) -> (x-y=w1668:dbl)
          n570 = Subtract(x=w1639, y=w1636) -> (x-y=w1635:dbl)
          n571 = Add(x=w1613, y=w1746) -> (x+y=w1745:i32[])
          n572 = Square Root(x=w1668) -> (sqrt(x)=w1666:dbl)
          n573 = local read "veränderte Methode benutzen"() -> (w1599:bool)
          n574 = Square Root(x=w1635) -> (sqrt(x)=w1633:dbl)
          n575 = Add(x=w1667, y=w1666) -> (x+y=w1664:dbl)
          n576 = local read "Methodenwechsel?"() -> (w1754:bool)
          n577 = Add(x=w1634, y=w1633) -> (x+y=w1597:dbl)
          n578 = To Fixed-Point(fixed-point type=fxp<+/-,16,4> 0.0 ("USetp [V]Mach1"), number=w1664) -> (fixed-point=w1661:fxp<+/-,16,4>)
          n579 = global read "gvbooleschRT.vi" "global stop RT"() -> (w1755:bool)
          n580 = To Fixed-Point(fixed-point type=fxp<+/-,16,4> 0.0 ("USetp [V]Mach1"), number=w1597) -> (fixed-point=w1623:fxp<+/-,16,4>)
          n581 = Or(x=w1754, y=w1755) -> (x .or. y?=w1600:bool)
          n582 = Or(x=w1600, y=w1599) -> (x .or. y?=w1598:bool)
          n583 = xnode "Read/Write Control"("FPGA VI Reference In"=w1660, "USetp[V]Mach1"=w1661, "USetp[V]Mach2"=w1623) -> ()  [unwired: 1 in, 2 out]
        }
        n584 = Equal?(x=w1592, y=0) -> (x = y?=w1590:bool)
        n585 = while "Zeit" {
          tunnel: w1590 -> [w2085]
          tunnel: [w2079] -> w1589
          tunnel: w1588 -> [w2084]
          tunnel: [w2072] -> w1587
          tunnel: w1584 -> [w2073]
          tunnel: w1566 -> [w2081]
          i -> [w2088]
          stop <- w2068 stop-if-true
          n586 = Equal?(x=w2088, y=0) -> (x = y?=w2086:bool)
          n587 = call "Warten3"("Count(mSec)"=u32 50) -> ()  [unwired: 1 out]
          n588 = And(x=w2085, y=w2086) -> (x .and. y?=w2090:bool)
          n589 = xnode "Elapsed Timer"("reset"=w2090) -> ("elapsed time (ms)"=w2093:i32)  [unwired: 2 in, 1 out]
          n590 = local read "veränderte Methode benutzen"() -> (w2070:bool)
          n591 = local read "Methodenwechsel?"() -> (w2083:bool)
          n592 = global read "gvbooleschRT.vi" "global stop RT"() -> (w2082:bool)
          n593 = Or(x=w2083, y=w2082) -> (x .or. y?=w2069:bool)
          n594 = To Double Precision Float(number=w2093) -> (double precision float=w2092:dbl)
          n595 = Or(x=w2070, y=w2069) -> (x .or. y?=w2068:bool)
          n596 = Divide(x=w2092, y=1000.0) -> (x/y=w2079:dbl)
          "Big Ben" <- w2079
          n597 = Subtract(x=w2079, y=w2084) -> (x-y=w2078:dbl)
          "Methodenzeit" <- w2078
          n598 = for {
            tunnel: w2081 -> [w2096] mode=indexing
            tunnel: w2078 -> [w2097]
            tunnel: [w2095] -> w2080 mode=indexing
            tunnel: [w2094] -> w2077 mode=indexing
            n599 = Quotient & Remainder(x=w2097, y=w2096) -> (x-y*floor(x/y)=w2095:dbl, floor(x/y)=w2094:dbl)
          }
          "Zykluszeiten 0, 1, 2A, 2B" <- w2080
          n600 = Build Array (concatenate)(w2079, w2078, w2080) -> (w2071:dbl[])
          n601 = To Long Integer(number=w2077) -> (32bit integer=w2076:i32[])
          "Zyklusnummern 0, 1, 2A, 2B" <- w2076
          n602 = local write "Big Ben, Methodenzeit, Zykluszeit0, Zykluszeit1, Zykluszeit2A, Zykluszeit2B"(w2071) -> ()
          n603 = Index Array(array=w2076, index=1 ("Index")) -> (element=w2074:i32)
          n604 = Add(x=w2074, y=w2073) -> (x+y=w2072:i32)
          "Zyklnum1ges" <- w2072
        }
        n605 = global read "gvbooleschRT.vi" "global stop RT"() -> (w1593:bool)
      }
      n606 = while {
        tunnel: w361 -> [w588]
        stop <- w592 stop-if-true
        n607 = local read "Mod1Mod2Mod3/AITrapsMachs1Hz"() -> (w581:dbl[])
        n608 = local read "Zyklusnummern 0, 1, 2A, 2B"() -> (w584:i32[])
        n609 = local read "Big Ben, Methodenzeit, Zykluszeit0, Zykluszeit1, Zykluszeit2A, Zykluszeit2B"() -> (w582:dbl[])
        n610 = local read "MFC1A Integriert"() -> (w579:dbl)
        n611 = local read "Zyklnum1ges"() -> (w586:i32)
        n612 = local read "MWHorst"() -> (w580:dbl[])
        n613 = To Double Precision Float(number=w586) -> (double precision float=w585:dbl)
        n614 = To Double Precision Float(number=w584) -> (double precision float=w583:dbl[])
        n615 = local read "aktuelle TDMS-Datei"() -> (w589:refnum<k34>)
        n616 = call "Warten20"("Count(mSec)"=u32 1000) -> ()  [unwired: 1 out]
        n617 = Build Array (concatenate)(w585, w583, w582, w581, w580, w579) -> (w587:dbl[])
        n618 = TDMS Write(0:w589, 1:enum16{"decimated", "interleaved"}."interleaved" ("Daten-Layout (0:dezimiert)"), 7:w588, 9:w587) -> ()  [unwired: 2 in, 4 out]
        n619 = global read "gvbooleschRT.vi" "global stop RT"() -> (w592:bool)
      }
      n620 = while {
        stop <- w612 stop-if-true
        n621 = call "Warten17"("Count(mSec)"=u32 1000 ("Zu wartende ms")) -> ()  [unwired: 1 out]
        n622 = Get Date/Time In Seconds() -> (seconds since 1Jan1904=w614:timestamp)
        n623 = Format Date/Time String(time format string (%c)="%Y%m%d%H%M%S" ("Zeitformatierungs-String (%c)"), seconds (now)=w614) -> (date/time string=→"Datum/Zeit":string)  [unwired: 1 in]
        n624 = global read "gvbooleschRT.vi" "global stop RT"() -> (w612:bool)
      }
      n625 = while {
        tunnel: w394 -> [w708]
        tunnel: w355 -> [w709]
        shift-right: [w707] -> _
        shift-left: w352 -> [w710]
        shift-right: [w706] -> _
        shift-left: 0 ("Zähler serielle Kommunikation") -> [w705]
        stop <- w703 stop-if-true
        n626 = call "Warten10"("Count(mSec)"=u32 100) -> ()  [unwired: 1 out]
        n627 = local read "Zähler serielle Kommunikation"() -> (w706:i32)
        n628 = Not Equal?(x=w706, y=w705) -> (x != y?=w704:bool)
        n629 = case shown="True" w704 {
          tunnel: w710 -> [w711 w716]
          tunnel: w709 -> [_ w715]
          tunnel: w708 -> [_ w714]
          tunnel: [w711 w712] -> w707
          frame False {
          }
          frame True {
            n630 = local read "RS-232"() -> (w713:string)
            n631 = for {
              tunnel: w713 -> [w731]
              tunnel: w714 -> [w729] mode=indexing
              tunnel: w715 -> [w728] mode=indexing
              shift-right: [w726] -> w712
              shift-left: w716 -> [w725]
              i -> [w727]
              n632 = Match Pattern(string=w731, regular expression=w729) -> (match substring=w730:string, after substring=w721:string)  [unwired: 1 in, 2 out]
              n633 = Equal?(x=w730, y=w729) -> (x = y?=w719:bool)
              n634 = String Subset(string=w721, length (rest)=4 ("Länge (Rest)")) -> (substring=w720:string)  [unwired: 1 in]
              n635 = for {
                N: 4 -> [_]
                tunnel: w720 -> [w744]
                shift-right: [w732] -> w718
                shift-left: TRUE -> [w733]
                i -> [w743]
                n636 = String Subset(string=w744, offset (0)=w743, length (rest)=1 ("Länge (Rest)")) -> (substring=w739:string)
                n637 = Equal?(x=w739, y="0") -> (x = y?=w740:bool)
                n638 = Hexadecimal String To Number(string=w739, default (0uL)=0.0) -> (number=w737:dbl)  [unwired: 1 in, 1 out]
                n639 = Greater?(x=w737, y=0.0) -> (0:w735:bool)
                n640 = Or(x=w740, y=w735) -> (x .or. y?=w734:bool)
                n641 = And(x=w733, y=w734) -> (x .and. y?=w732:bool)
              }
              n642 = And(x=w719, y=w718) -> (x .and. y?=w717:bool)
              n643 = case shown="True" w717 {
                tunnel: w720 -> [_ w746]
                tunnel: w728 -> [_ w752]
                tunnel: w727 -> [_ w749]
                tunnel: [w745 w748] -> w726
                tunnel: w725 -> [w745 w747]
                frame False {
                }
                frame True {
                  n644 = Hexadecimal String To Number(string=w746, default (0uL)=0.0) -> (number=w751:dbl)  [unwired: 1 in, 1 out]
                  n645 = Multiply(x=w752, y=w751) -> (x*y=w750:dbl)
                  n646 = Replace Array Subset(array=w747, new element=w750, index=w749) -> (w748:dbl[])
                }
              }
            }
            "MWHorst" <- w712
          }
        }
        n647 = global read "gvbooleschRT.vi" "global stop RT"() -> (w703:bool)
      }
      n648 = while {
        tunnel: path "c:/fromcriocmd.txt" ("Dateipfad (Dialog verwenden)") -> [w623]
        tunnel: w367 -> [w624]
        stop <- w625 stop-if-true
        n649 = local read "Dateien fürs MS schicken?"() -> (w622:bool)
        n650 = global read "gvbooleschRT.vi" "global stop RT"() -> (w621:bool)
        n651 = Not(x=w621) -> (.not. x?=w620:bool)
        n652 = Boolean To (0,1)(Boolean=w620) -> (0, 1=w618:i16)
        n653 = case shown="True" w622 {
          tunnel: w623 -> [_ w632]
          tunnel: w624 -> [_ w631]
          tunnel: w623 -> [_ w628]
          frame False {
          }
          frame True {
            n654 = flat-sequence {
              tunnel: w628 -> [w634]
              tunnel: w632 -> [w635]
              tunnel: [w635] -> w627
              tunnel: [w634] -> w626
              tunnel: [w675] -> w629
              tunnel: w627 -> [w675]
              tunnel: w626 -> [w636]
              tunnel: [w682] -> w630
              tunnel: w629 -> [w687]
              tunnel: w631 -> [w695]
              tunnel: w630 -> [w691]
              frame #0 {
                n655 = call "Warten14"("Count(mSec)"=u32 1000 ("Zu wartende ms")) -> ()  [unwired: 1 out]
              }
              frame #1 {
                n656 = Open/Create/Replace File(file path (use dialog)=w636, operation (0:open)=T6."open" ("Operation (0:Öffnen)")) -> (refnum out=w640:refnum<file>)  [unwired: 4 in, 2 out]
                n657 = Read from Text File(file (use dialog)=w640) -> (refnum out=w641:refnum<file>)  [unwired: 3 in, 3 out]
                n658 = local read "Datum/Zeit"() -> (w663:string)
                n659 = Set File Position(offset (in bytes) (0)=i64 5 ("Offset (in Byte) (0)"), refnum=w641) -> (refnum out=w648:refnum<file>)  [unwired: 2 in, 1 out]
                n660 = local read "Zyklnum1ges"() -> (w665:i32)
                n661 = Write to Text File(file (use dialog)=w648, text=w663) -> (refnum out=w650:refnum<file>)  [unwired: 2 in, 2 out]
                n662 = Set File Position(offset (in bytes) (0)=i64 27 ("Offset (in Byte) (0)"), refnum=w650) -> (refnum out=w649:refnum<file>)  [unwired: 2 in, 1 out]
                n663 = Format Value(format string="%03d" ("Format-String"), value (0)=w665) -> (output string=w667:string)  [unwired: 1 in]
                n664 = String Length(string="Info") -> (length=w668:i32)
                n665 = Write to Text File(file (use dialog)=w649, text=w667) -> (refnum out=w651:refnum<file>)  [unwired: 2 in, 2 out]
                n666 = Subtract(x=100, y=w668) -> (x-y=w670:i32)
                n667 = Initialize Array(" ", w670) -> (w672:string[])
                n668 = Set File Position(offset (in bytes) (0)=i64 37 ("Offset (in Byte) (0)"), refnum=w651) -> (refnum out=w652:refnum<file>)  [unwired: 2 in, 1 out]
                n669 = Concatenate Strings("Info", w672) -> (w674:string)
                n670 = Write to Text File(file (use dialog)=w652, text=w674) -> (refnum out=w653:refnum<file>)  [unwired: 2 in, 2 out]
                n671 = Set File Position(offset (in bytes) (0)=i64 196 ("Offset (in Byte) (0)"), refnum=w653) -> (refnum out=w654:refnum<file>)  [unwired: 2 in, 1 out]
                n672 = case shown="0, Default" "wie wird gespeichert?" {
                  tunnel: ["Time" "Cycle" "all"] -> w662
                  tunnel: [i64 209 ("Größe (in Byte)") i64 210 ("Größe (in Byte)") i64 208 ("Größe (in Byte)")] -> w655
                  frame 0, Default {
                  }
                  frame 1 {
                  }
                  frame 2 {
                  }
                }
                n673 = Write to Text File(file (use dialog)=w654, text="Speicherlänge") -> (refnum out=w660:refnum<file>)  [unwired: 2 in, 2 out]
                n674 = Set File Position(offset (in bytes) (0)=i64 205 ("Offset (in Byte) (0)"), refnum=w660) -> (refnum out=w659:refnum<file>)  [unwired: 2 in, 1 out]
                n675 = Write to Text File(file (use dialog)=w659, text=w662) -> (refnum out=w661:refnum<file>)  [unwired: 2 in, 2 out]
                n676 = Set File Size(6:w655, 7:w661) -> (3:w656:refnum<file>)  [unwired: 1 in, 1 out]
                n677 = Set File Position(offset (in bytes) (0)=i64 0 ("Offset (in Byte) (0)"), refnum=w656) -> (refnum out=w646:refnum<file>)  [unwired: 2 in, 1 out]
                n678 = Read from Text File(file (use dialog)=w646) -> (refnum out=w657:refnum<file>, text=→"Text 6":string)  [unwired: 3 in, 2 out]
                n679 = Close File(refnum=w657) -> ()  [unwired: 1 in, 2 out]
              }
              frame #2 {
                n680 = call "Warten16"("Count(mSec)"=u32 500 ("Zu wartende ms")) -> ()  [unwired: 1 out]
                n681 = call <vilib>:"FTP Put File.vi"("remote port (21)"=u16 21, "password"="1" ("user"), "binary (F)"=TRUE, "user"="1", "local path"=w687, "remote path"="fromcriocmd.txt", "host"="10.1.1.101") -> ("error out"=w682:errorcluster)  [unwired: 3 in, 1 out]
              }
              frame #3 {
                n682 = call <vilib>:"FTP Put File.vi"("remote port (21)"=u16 21, "password"="1" ("user"), "binary (F)"=TRUE, "user"="1", "error in (no error)"=w691, "local path"=w695, "remote path"="fromcriordy.txt", "host"="10.1.1.101") -> ()  [unwired: 2 in, 2 out]
              }
            }
          }
        }
        n683 = To Unsigned Long Integer(number=w618) -> (unsigned 32bit integer=w617:u32)
        n684 = Multiply(x=u32 10000 ("Zu wartende ms"), y=w617) -> (x*y=w616:u32)
        n685 = call "Warten11"("Count(mSec)"=w616) -> ()  [unwired: 1 out]
        n686 = global read "gvbooleschRT.vi" "global stop RT"() -> (w625:bool)
      }
      n687 = while {
        shift-right: [w2139] -> w416
        shift-left: w419 -> [w2141]
        shift-right: [w2138] -> w415
        shift-left: w418 -> [w2140]
        shift-right: [w2142] -> _
        shift-left: 0 ("Zyklusnummer1") -> [w2144]
        tunnel: w366 -> [w2137]
        tunnel: w365 -> [w2136]
        stop <- w2146 stop-if-true
        n688 = call "Warten2"("Count(mSec)"=u32 500) -> ()  [unwired: 1 out]
        n689 = local read "Zyklnum1ges"() -> (w2142:i32)
        n690 = Greater?(x=w2142, y=w2144) -> (0:w2143:bool)
        n691 = case shown="True" w2143 {
          tunnel: w2142 -> [_ w2152]
          tunnel: w2141 -> [w2148 w2157]
          tunnel: w2140 -> [w2147 w2156]
          tunnel: [w2148 w2153] -> w2139
          tunnel: [w2147 w2151] -> w2138
          tunnel: w2137 -> [_ w2150]
          tunnel: w2136 -> [_ w2149]
          frame False {
          }
          frame True {
            n692 = flat-sequence {
              tunnel: w2157 -> [w2159]
              tunnel: w2156 -> [w2158]
              tunnel: [w2159] -> w2155
              tunnel: [w2158] -> w2154
              tunnel: w2155 -> [w2175]
              tunnel: w2154 -> [w2176]
              tunnel: [w2176] -> w2153
              tunnel: w2152 -> [w2170]
              tunnel: [w2168] -> w2151
              tunnel: w2150 -> [w2161]
              tunnel: w2149 -> [w2160]
              frame #0 {
                "aktuelle TDMS-Datei" <- w2158
              }
              frame #1 {
                n693 = TDMS Close(11:w2175) -> ()  [unwired: 1 in, 2 out]
                n694 = local read "Methodennummer"() -> (w2165:i32)
                n695 = Add(x=w2170, y=1) -> (x+y=w2172:i32)
                n696 = Number To Decimal String(number=w2165) -> (decimal integer string=w2164:string)  [unwired: 1 in]
                n697 = Number To Decimal String(number=w2172) -> (decimal integer string=w2162:string)  [unwired: 1 in]
                n698 = Concatenate Strings(w2161, "m", w2164, "z", w2162, ".tdms" ("String")) -> (w2171:string)
                n699 = Build Path(base path=w2160, name or relative path=w2171) -> (appended path=w2173:path)
                n700 = TDMS Open(10:T5."create" ("Operation (0:Öffnen)"), 11:w2173) -> (3:w2168:refnum<k34>)  [unwired: 4 in, 1 out]
              }
            }
          }
        }
        n701 = global read "gvbooleschRT.vi" "global stop RT"() -> (w2146:bool)
      }
      n702 = local read "Zyklnum1ges"() -> (w360:i32)
      n703 = while {
        shift-right: [w571] -> _
        shift-left: w360 -> [w574]
        shift-right: [w567] -> _
        shift-left: 0.0 -> [w569]
        stop <- w578 stop-if-true
        n704 = local read "MWHorst"() -> (w576:dbl[])
        n705 = local read "Zyklnum1ges"() -> (w571:i32)
        n706 = call "Warten22"("Count(mSec)"=u32 100) -> ()  [unwired: 1 out]
        n707 = Equal?(x=w574, y=w571) -> (x = y?=w573:bool)
        n708 = Index Array(array=w576, index=4 ("Index")) -> (element=w564:dbl)
        n709 = Boolean To (0,1)(Boolean=w573) -> (0, 1=w572:i16)
        n710 = Multiply(x=w564, y=3000.0) -> (x*y=w562:dbl)
        n711 = Divide(x=w562, y=64000.0) -> (x/y=w560:dbl)
        n712 = Divide(x=w560, y=600.0) -> (x/y=w565:dbl)
        n713 = To Double Precision Float(number=w572) -> (double precision float=w570:dbl)
        n714 = Multiply(x=w570, y=w569) -> (x*y=w568:dbl)
        n715 = global read "gvbooleschRT.vi" "global stop RT"() -> (w578:bool)
        n716 = Add(x=w565, y=w568) -> (x+y=w567:dbl)
        "MFC1A Integriert" <- w567
      }
    }
    frame #2 {
      n717 = TDMS Close(11:w2188) -> ()  [unwired: 1 in, 2 out]
      n718 = TDMS Close(11:w2187) -> ()  [unwired: 1 in, 2 out]
      n719 = local read "Ausgang"() -> (w2183:T2)
      n720 = xnode "Read/Write Control"("FPGA VI Reference In"=w2186, "global stop"=TRUE) -> ("FPGA VI Reference Out"=w2185:refnum<k20>)  [unwired: 1 in, 1 out]
      n721 = Build Array(w2183) -> (w2182:T1)
      n722 = local write "Eingang"(w2182) -> ()
      n723 = xnode "Close FPGA VI Reference"("FPGA VI Reference In"=w2185) -> ()  [unwired: 1 in, 1 out]
    }
  }
